vi "r3_Pick&Place_ladder_shih_v10_MPTv2.vi"() -> ()   [LabVIEW 2016]
uses:
  WTF is this.ctl
  Classes/Controllers/I-O/Copy of NI-DAQ Folder/NI-DAQ.lvclass
  D:/INTT/V1/Classes/Controllers/I-O/Copy of I-O Folder/I-O.lvclass
  Classes/Controllers/Dispenser/Copy of Ultimus V2 Folder/Ultimus V2.lvclass
  <vilib>/Analysis/coordinate.llb/2D Cartesian Coordinate Rotation (Scalar).vi
  <vilib>/Utility/file.llb/Read Delimited Spreadsheet (DBL).vi
  <vilib>/Utility/file.llb/Write Delimited Spreadsheet (DBL).vi
  Classes/Controllers/Motion/Copy of Motion Folder/Motion.lvclass
  Classes/Controllers/Camera/Copy of Controller Folder/Controller.lvclass
  <vilib>/Analysis/NI_AALPro.lvlib
  Classes/Controllers/I-O/Copy of I-O Folder/I-O.lvclass
panel:
  out "file indicator":dbl[][](array[numeric])
  out "?":dbl[](array[numeric]) format="%#_8g"
  in  "offset":dbl[](array[numeric])=[0.0, 0.0, 0.0, 0.0] format="%#_8g"
  out "HDI center positions":dbl[][](array[numeric]) format="%#_8g"
  out "HDI center positions":dbl[][](array[numeric])=[[459.92445114002015, 980.2358762511564, 78.77350133595746, 0.0015214873297426886]] format="%#_8g"
  out "CT sum up":dbl[](array[numeric])
  in  "txt switch":bool
  in  "MPT offset":dbl[][](array[numeric])=[[0.0, 0.0, 0.0, 0.0], [0.0, 0.0, 0.0, 0.0]] format="%#_8g"
  out "CT HPoS":dbl[][](array[numeric]) format="%#_8g"
  out "chip distance by OGP":dbl format="%#_8g"
  out "displacement":dbl[](array[numeric])
  out "gantry position test":dbl[](array[numeric])
  out "gantry target position":dbl[](array[numeric])
  out "chip distance by gantry":dbl format="%#_8g"
  out "after SL":dbl[](array[numeric]) format="%#_8g"
  out "after SR":dbl[](array[numeric]) format="%#_8g"
  out "after NL":dbl[](array[numeric]) format="%#_8g"
  out "S chip":dbl[](array[numeric]) format="%#_8g"
  out "N chip":dbl[](array[numeric]) format="%#_8g"
  in  "?":path=path "C:/Users/PAGANIS/Desktop/shih cheng wei/OGP/test1-2.txt"
  out "bless from OGP !!! Center of  stave":dbl[](array[numeric])
  out "bless from OGP !! measured stave size":dbl[](array[numeric])
  in  "Bless from OGP":bool
  out "FROM Detail !!! Center of module on stave":dbl[](array[numeric])
  out "FROM Detail !! measured stave size":dbl[](array[numeric])
  in  "Align Stave in detail":bool
  in  "check height?":bool=TRUE
  in  "Uttimus presssure":i64=10
  out "Status":bool
  out "measured HDI top-left position":dbl[][](array[numeric])
  in  "HDI vacuum channel":i32=18
  in  "vacuum":bool=TRUE
  in  "HDI vacuum":bool
  out "measured stave size":dbl[](array[numeric])
  out "Stave mark":dbl[][](array[numeric])
  out "Center of module on stave":dbl[](array[numeric])
  out "Measured HDI size":dbl[][](array[numeric])
  out "MPT positions on stave":T1[][](array[typedef]) format="%#_8g"
  in  "Default Stave dimension":dbl[](array[numeric])=[34.0, 472.0, -0.335295, -0.000320234]
  in  "Default Stave upper left mark":dbl[](array[numeric])=[584.376, 675.576, 70.9882, 0.000840064]
  out "Needle parking position":dbl[](array[numeric])
  in  "Uppler / Lower Stave":bool=TRUE
  out "Gantry current position":dbl[](array[numeric])
  in  "READ Position":bool
  in  "Needle Height Compenstation\n(glue gap)":dbl=0.33
  in  "Needle Alignment":bool
  in  "Parking position":dbl[](array[numeric])=[625.0, 625.0, 0.0, 0.01]
  in  "GOTO":bool
  in  "Default Pickup Tool Position":dbl[][](array[numeric])=[[166.21919, 608.63665, 49.475503, -0.0151898], [700.0, 800.0, 20.0, 0.01]]
  in  "deposit glue module":i32=1
  in  "Default HDI alignment \nmark position":dbl[](array[numeric])=[139.81, 893.561, 78.9867, 0.000191129]
  in  "Default HDI size":dbl[](array[numeric])=[24.2437, 231.446, -0.099339, 0.000191129]
  out "# of tasks excuted":i32
  out "PickupTool \nCenterPosition":dbl[](array[numeric]) format="%#_8g"
  in  "Inititalize":bool
  in  "Pick and place":bool
  in  "Deposit Glue":bool
  in  "Measure Pickup Tools":bool
  in  "Align Stave":bool
  out "default module position on stave":dbl[][](array[numeric])
  in  "Stop":bool
  in  "Measure HDI":bool
  # "Ladder Assembly"
  # "To switch the north/south\ntxt file \nswitch \noffset\nmodule pick up tool\nmodule direction"
  # "upper : north \nlower : south"
  # "Upper\nmodule"
  # "Lower\nmodule"
  # "Sensor 0.32 -> 200 micron glue thickness\nChips 0.37-> 140 micron glue thickness"
  # "ACTIONS"
  # "theta had *-1"
  # "Pick up tool and needle"
  # "Module infomation"
  # "Pick and Place"
  # "after assembly"
  # "CT"
  # "+"
  # "+"
  # "="
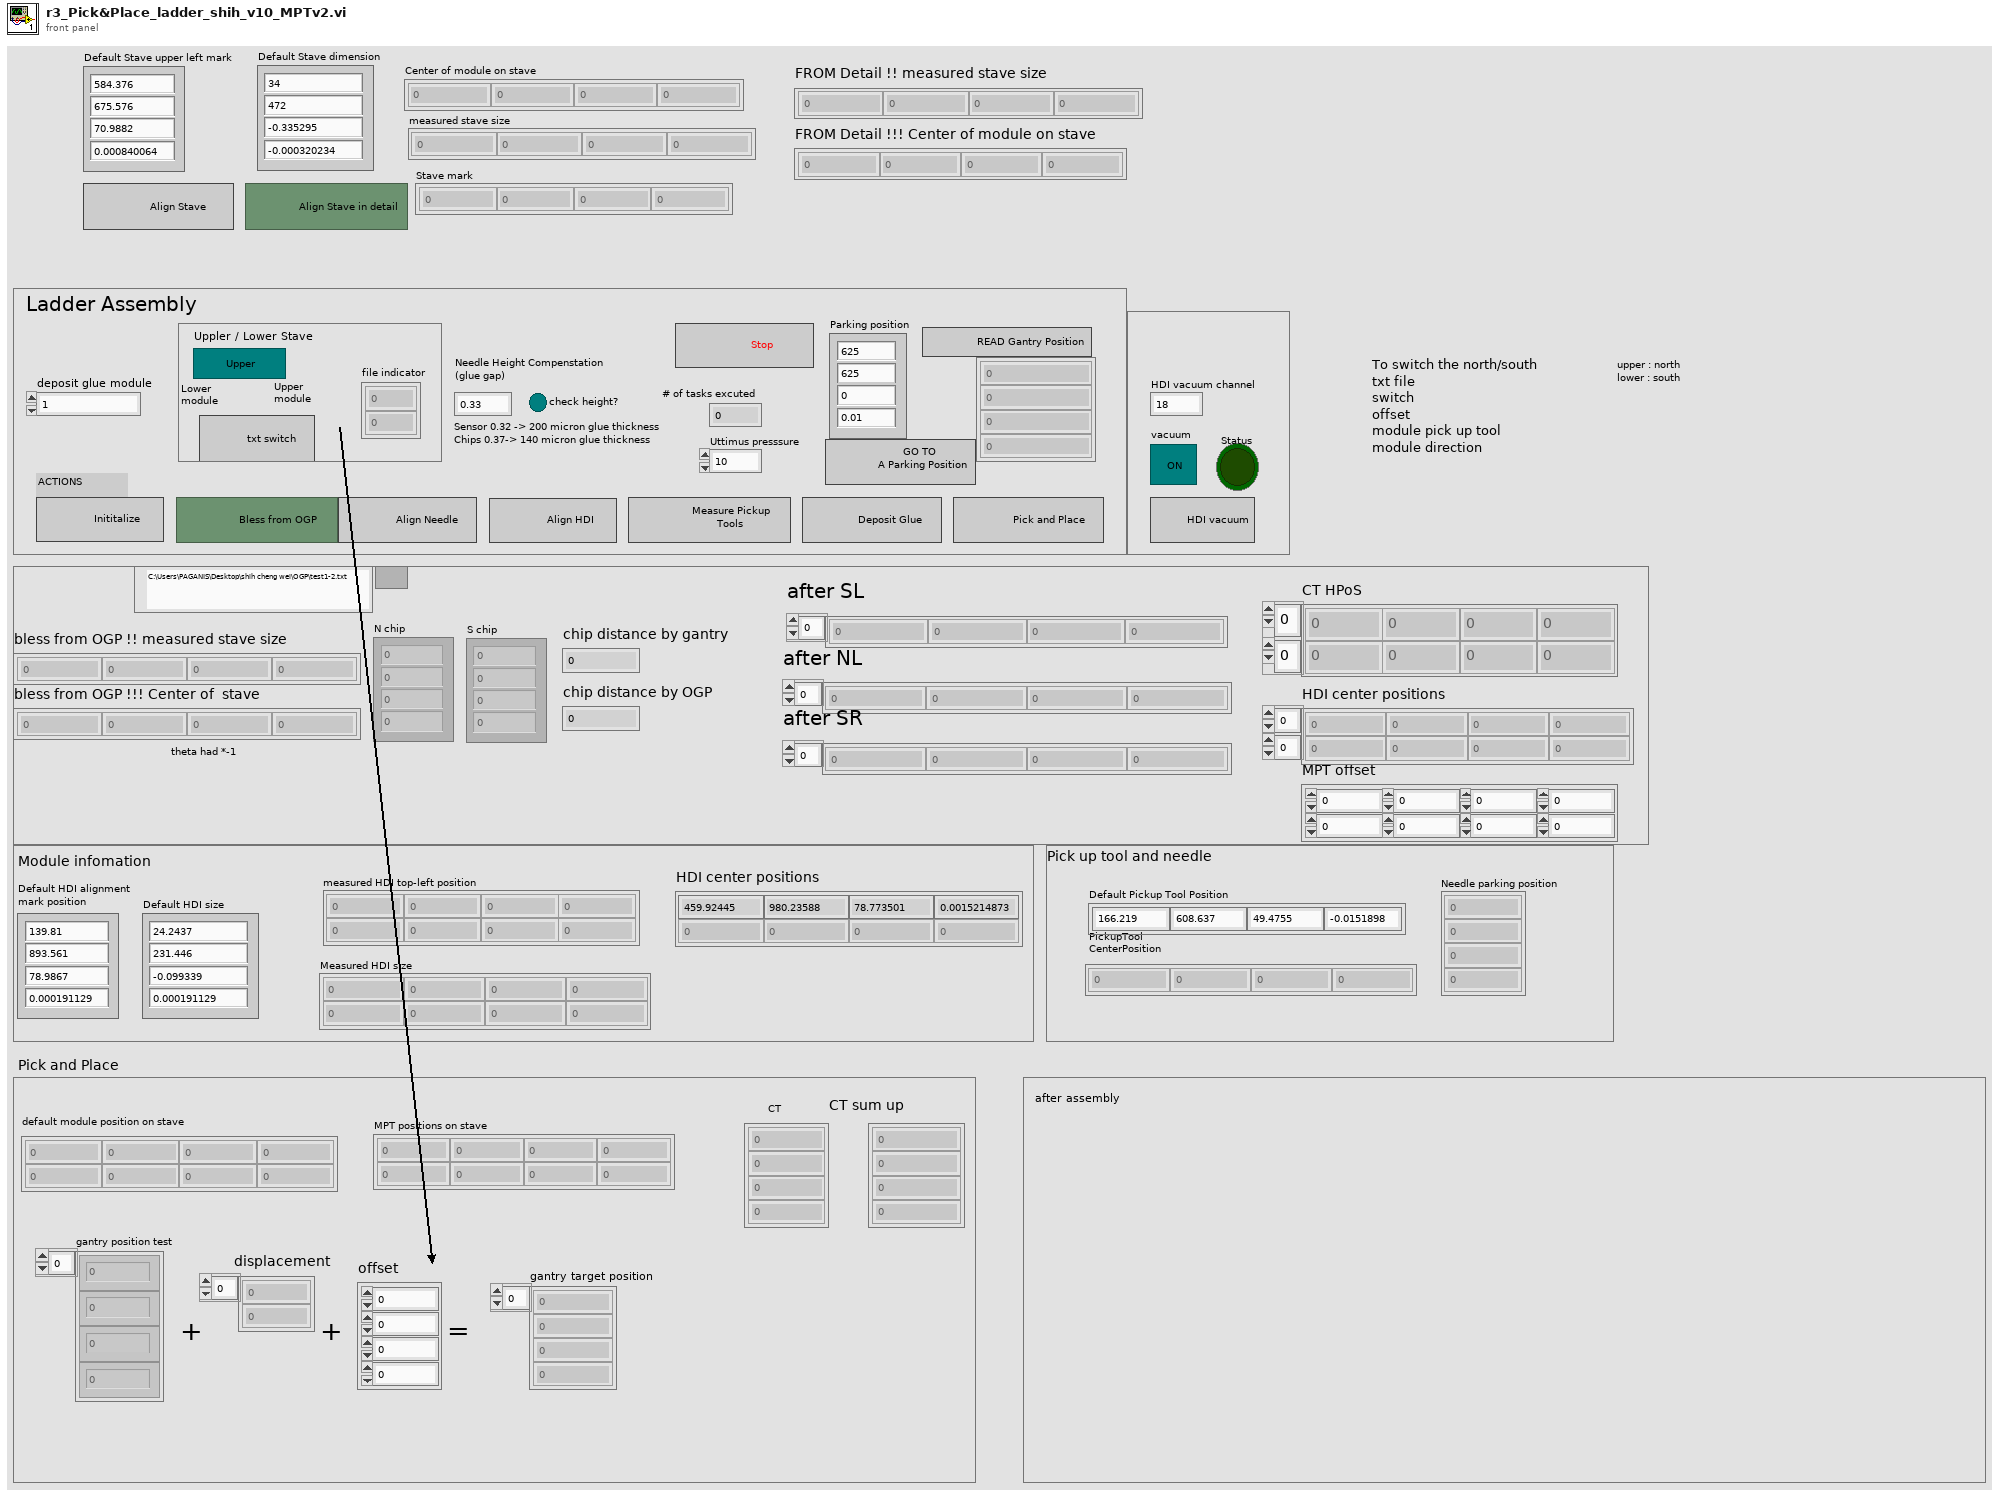
[diagram p1: front panel]
types:
  T1 = typedef "WTF is this.ctl" = dbl
  T2 = typedef "Controller.lvclass/Controllers.ctl" = cluster{"Copy of Motion.lvclass":refnum<class "Motion.lvclass">, "Copy of I-O.lvclass":refnum<class "I-O.lvclass">, "Copy of Dispenser.lvclass":refnum<class "Dispenser.lvclass">}
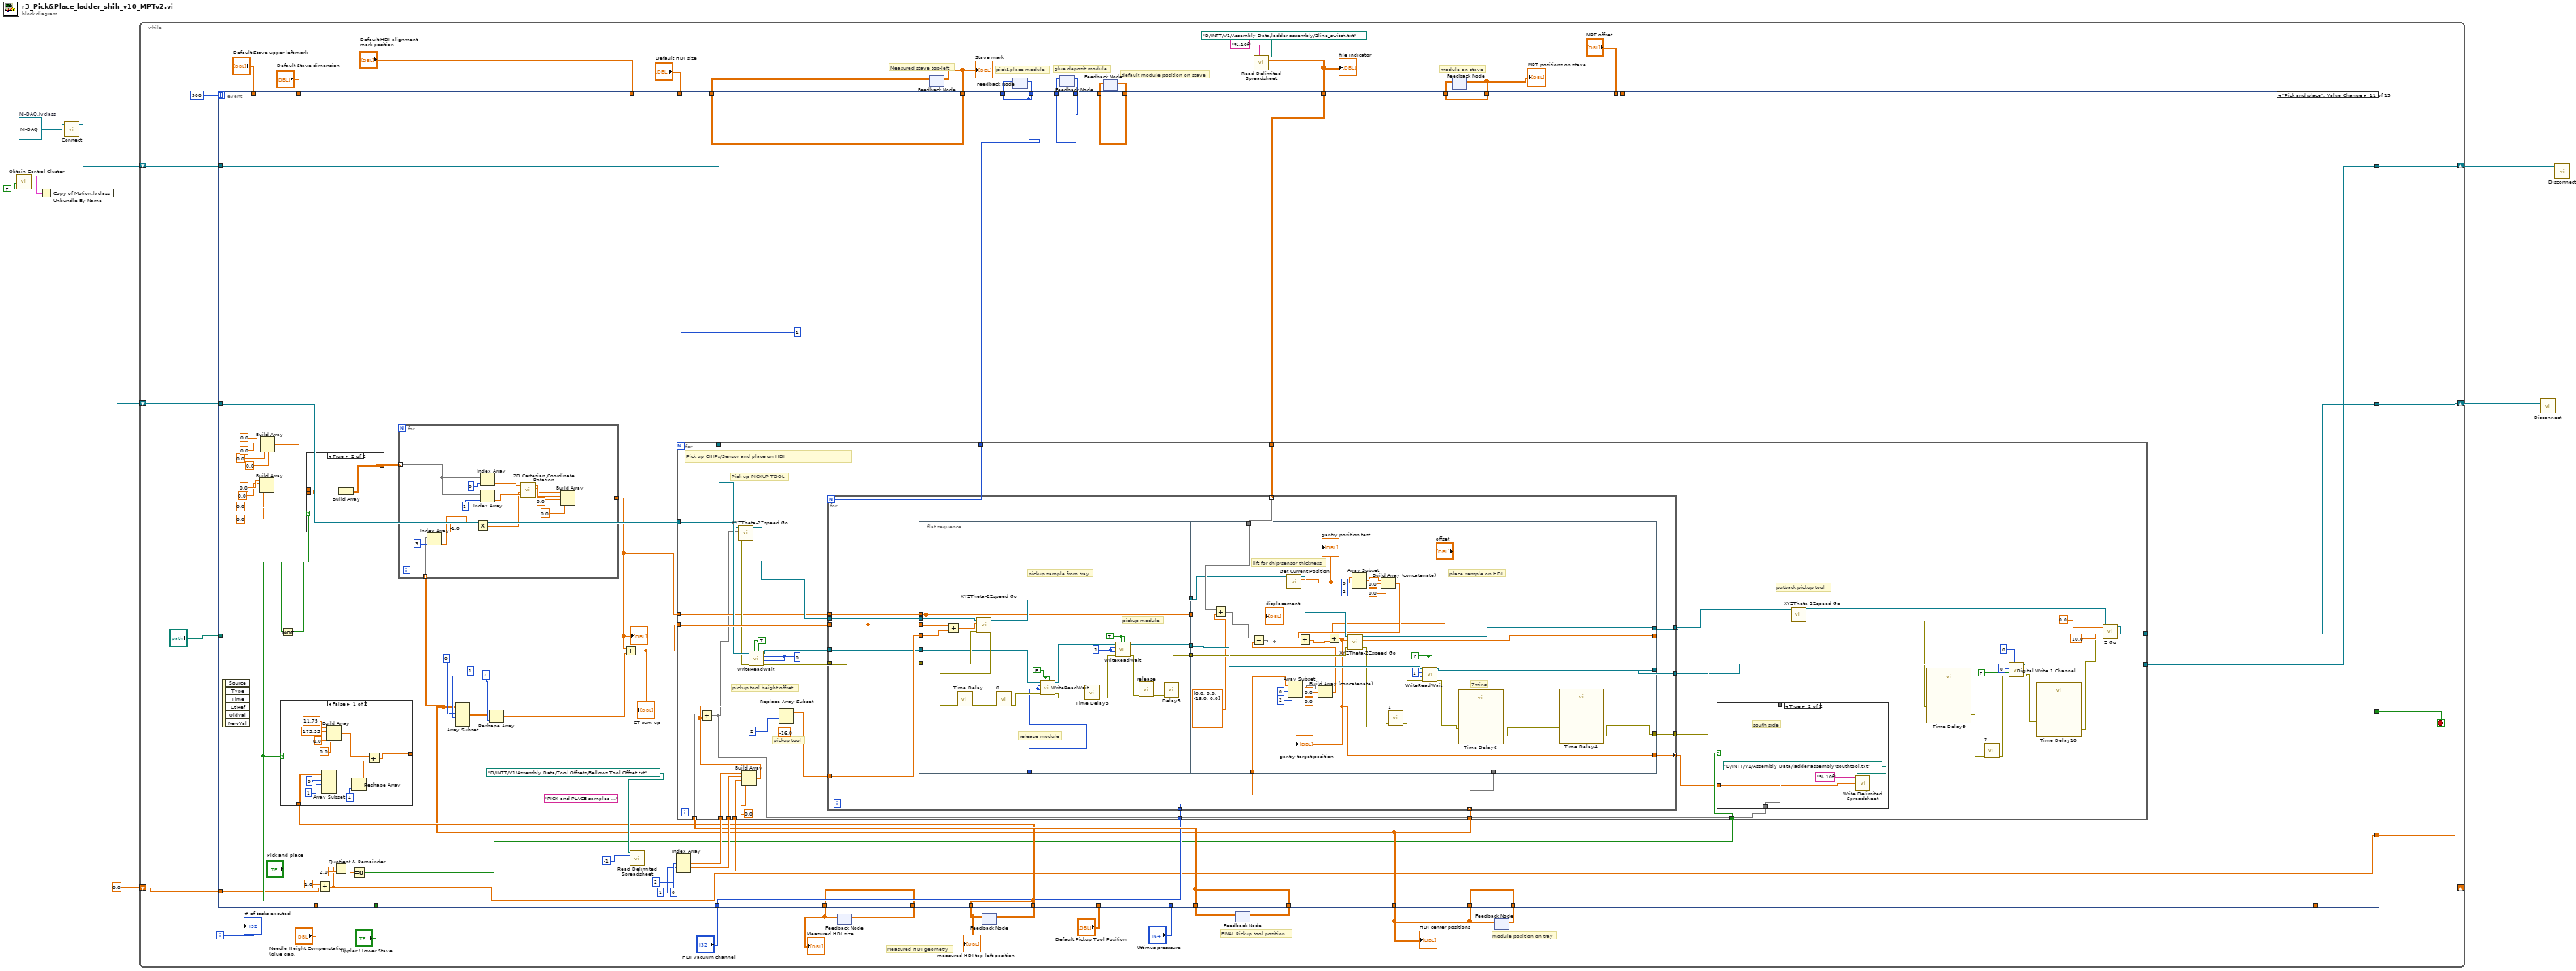
[diagram p0: block diagram]
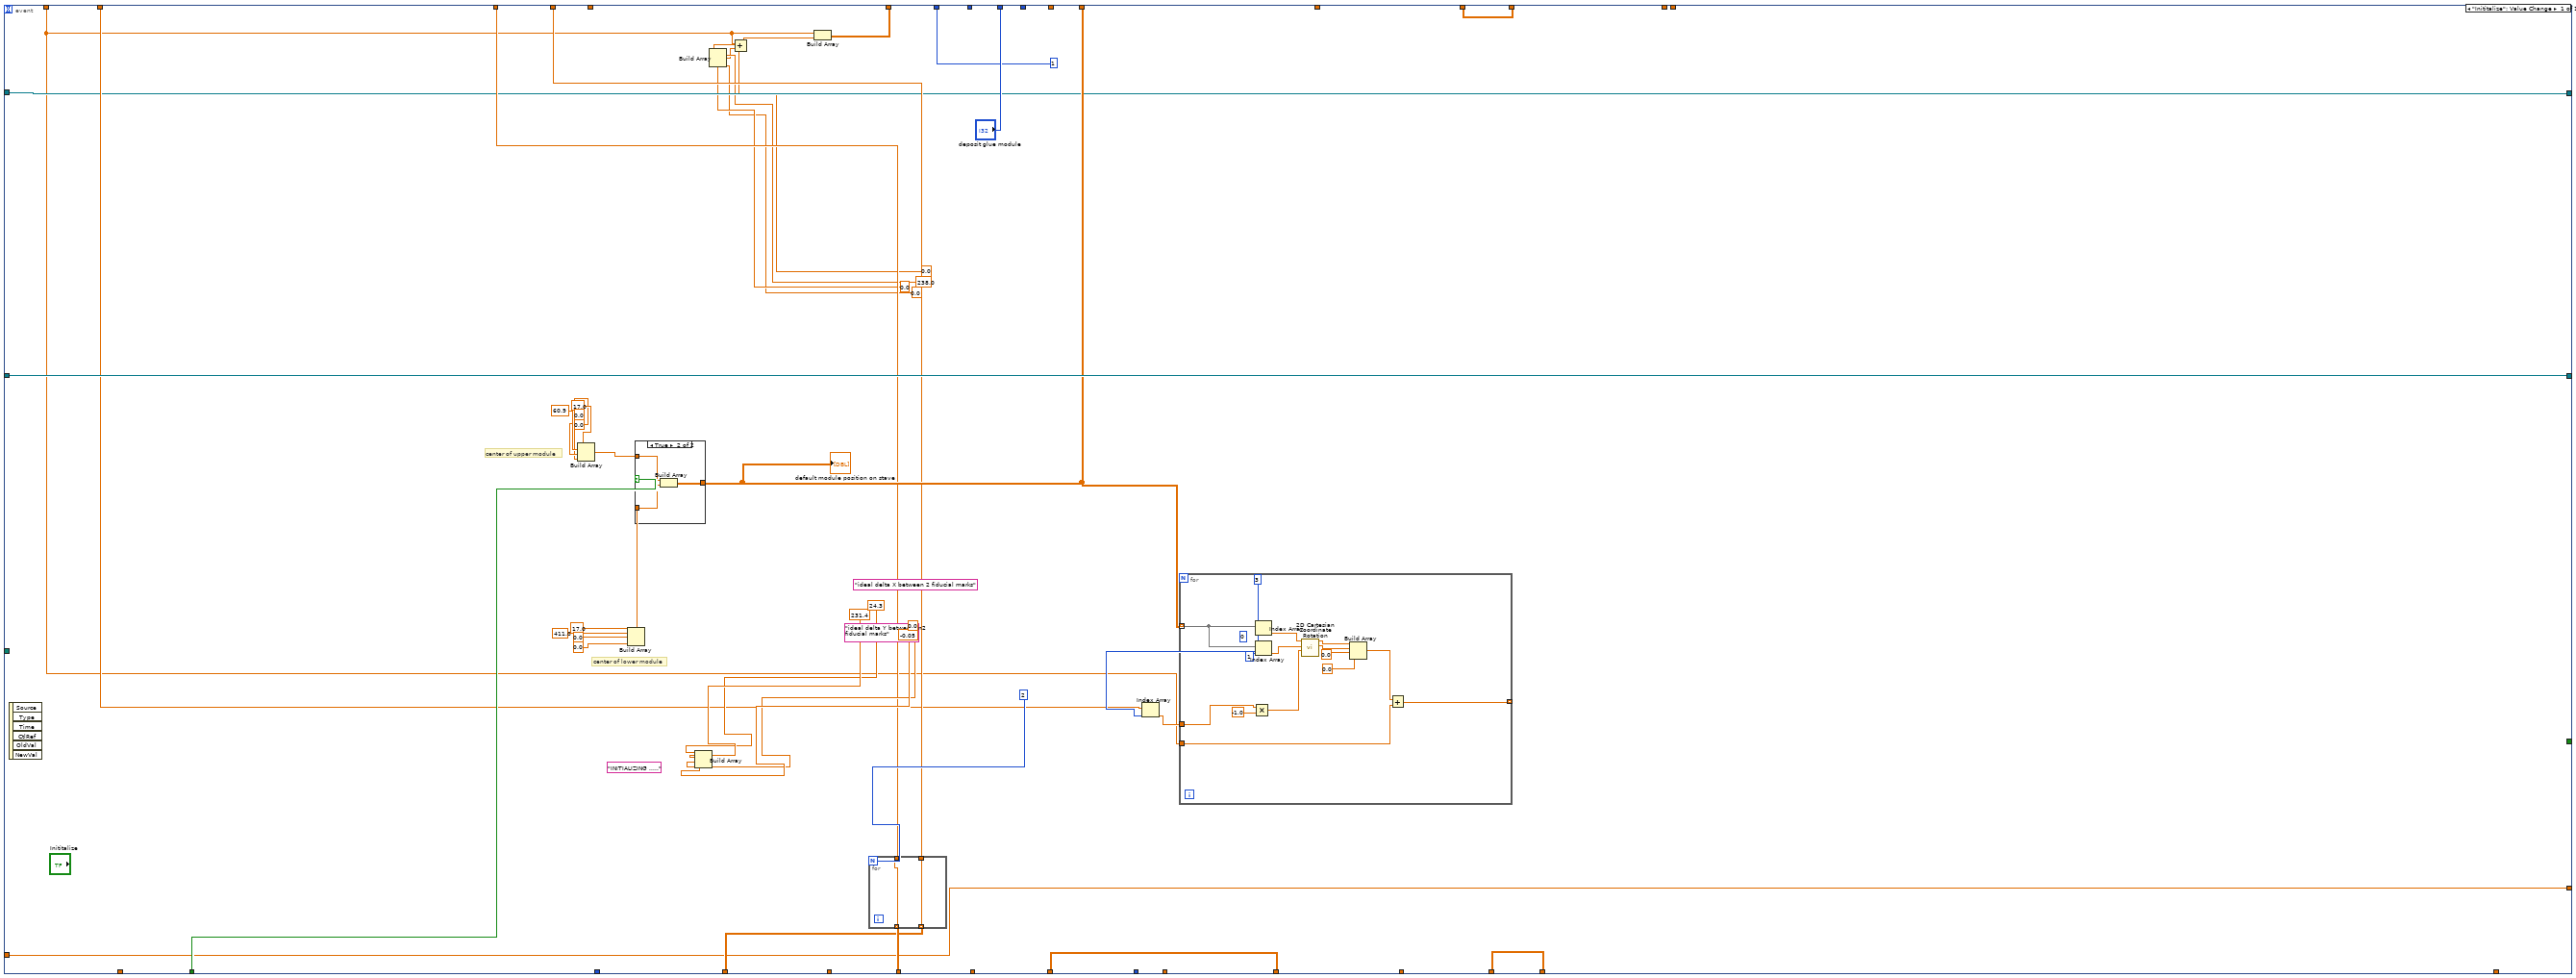
[diagram p2: hidden frame]
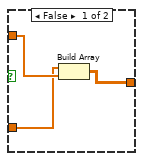
[diagram p3: hidden frame]
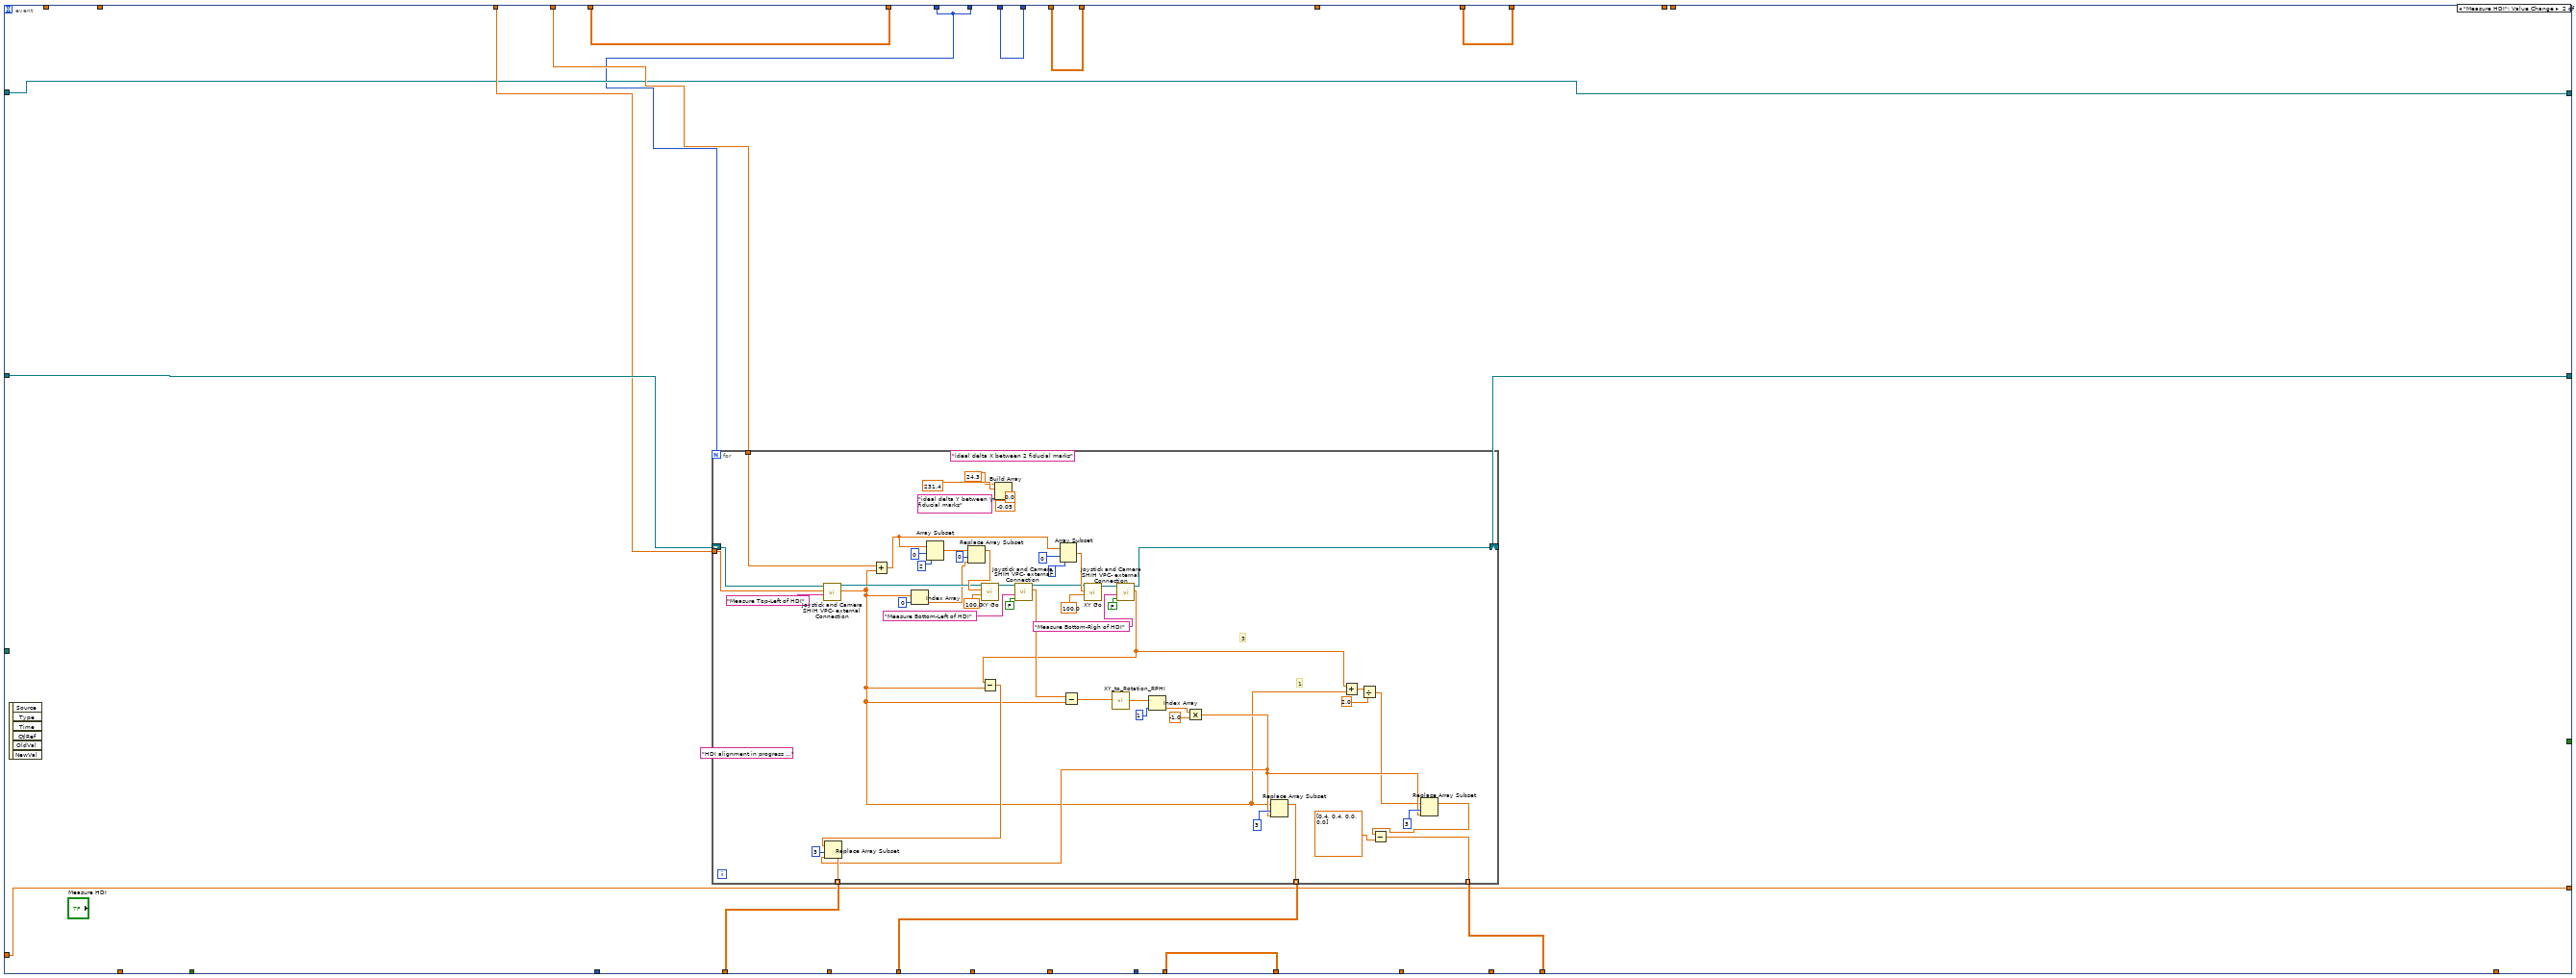
[diagram p4: hidden frame]
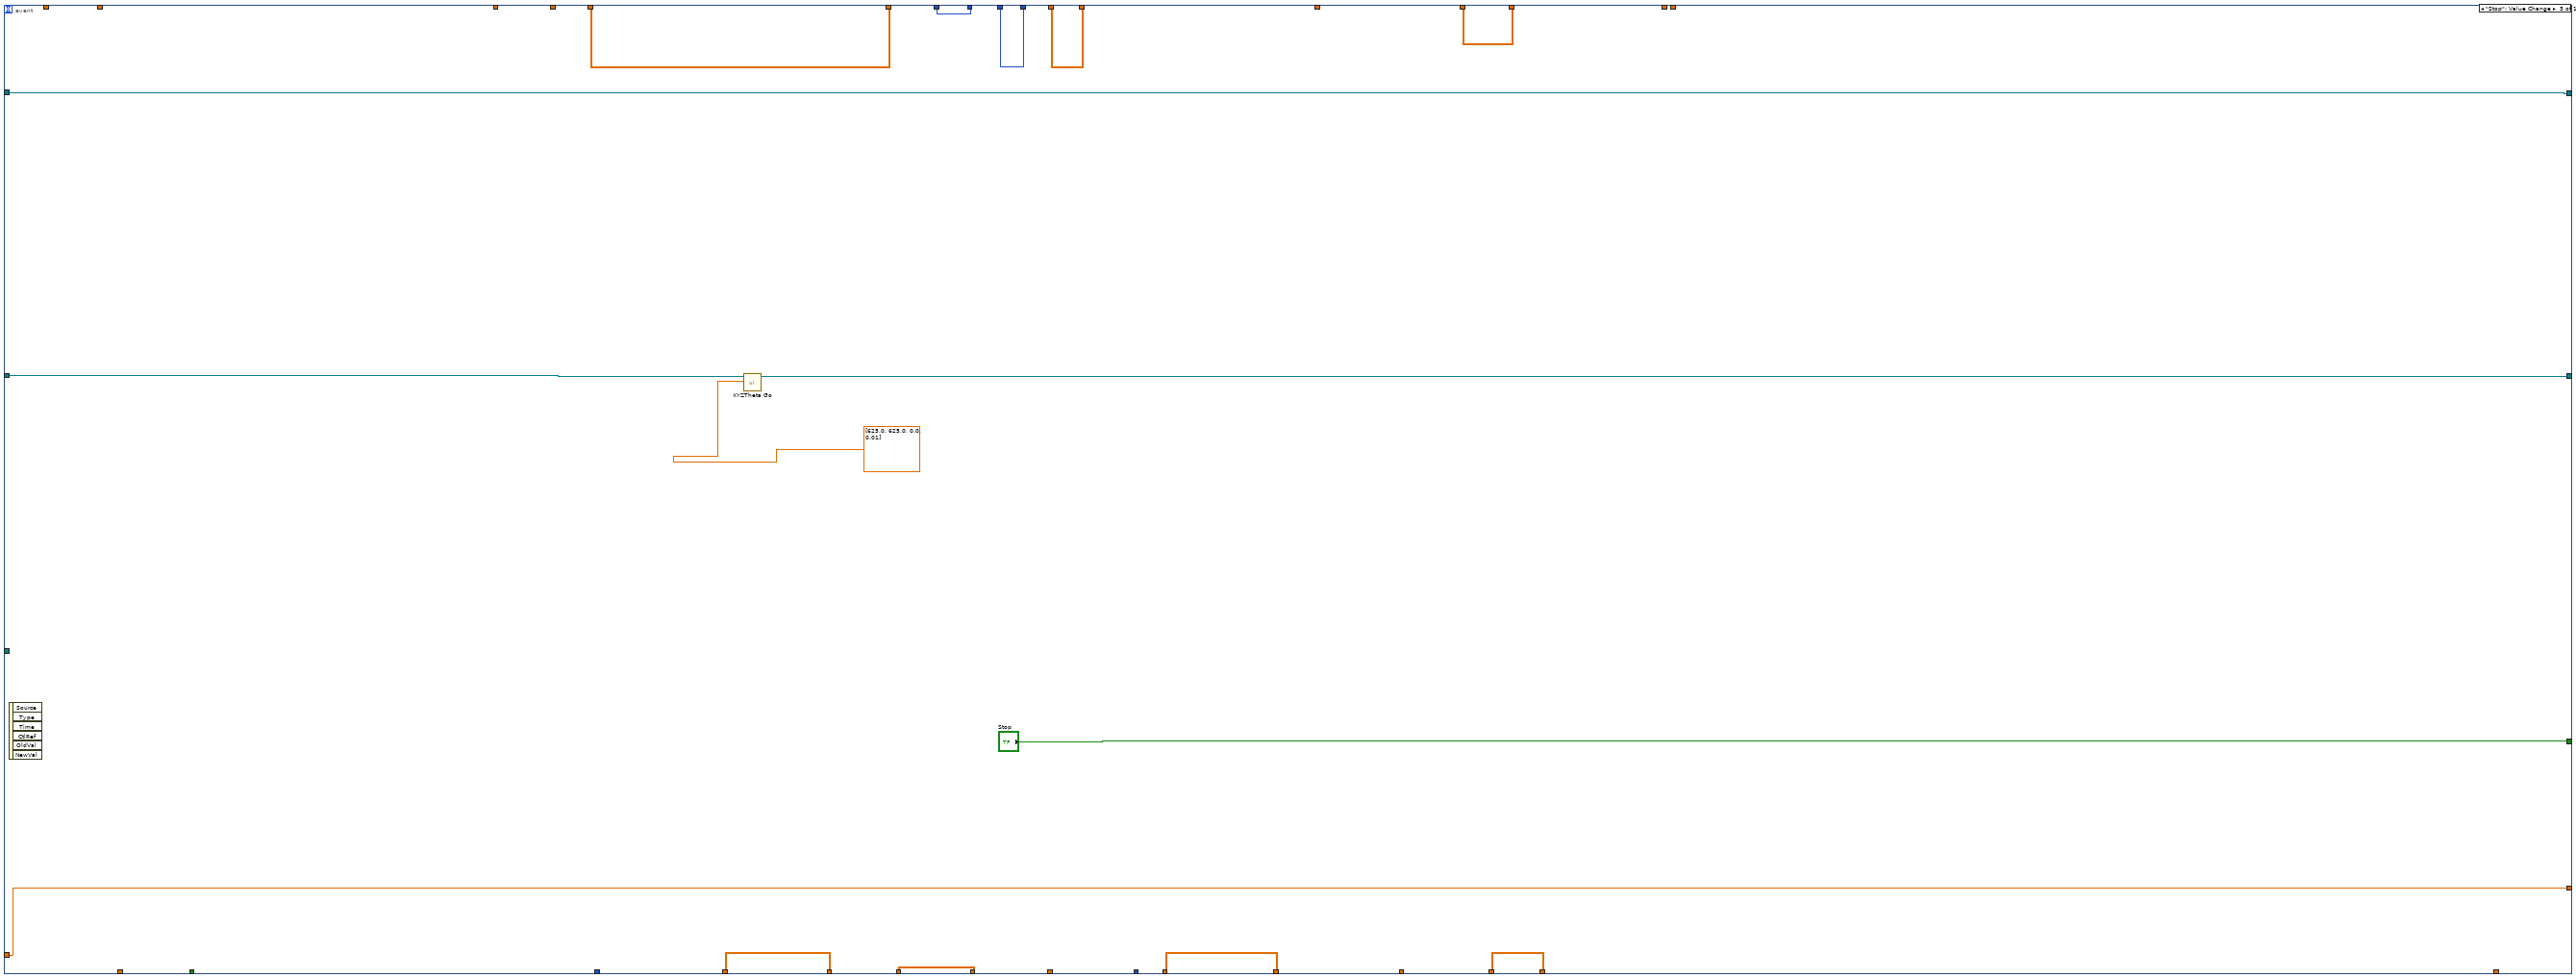
[diagram p5: hidden frame]
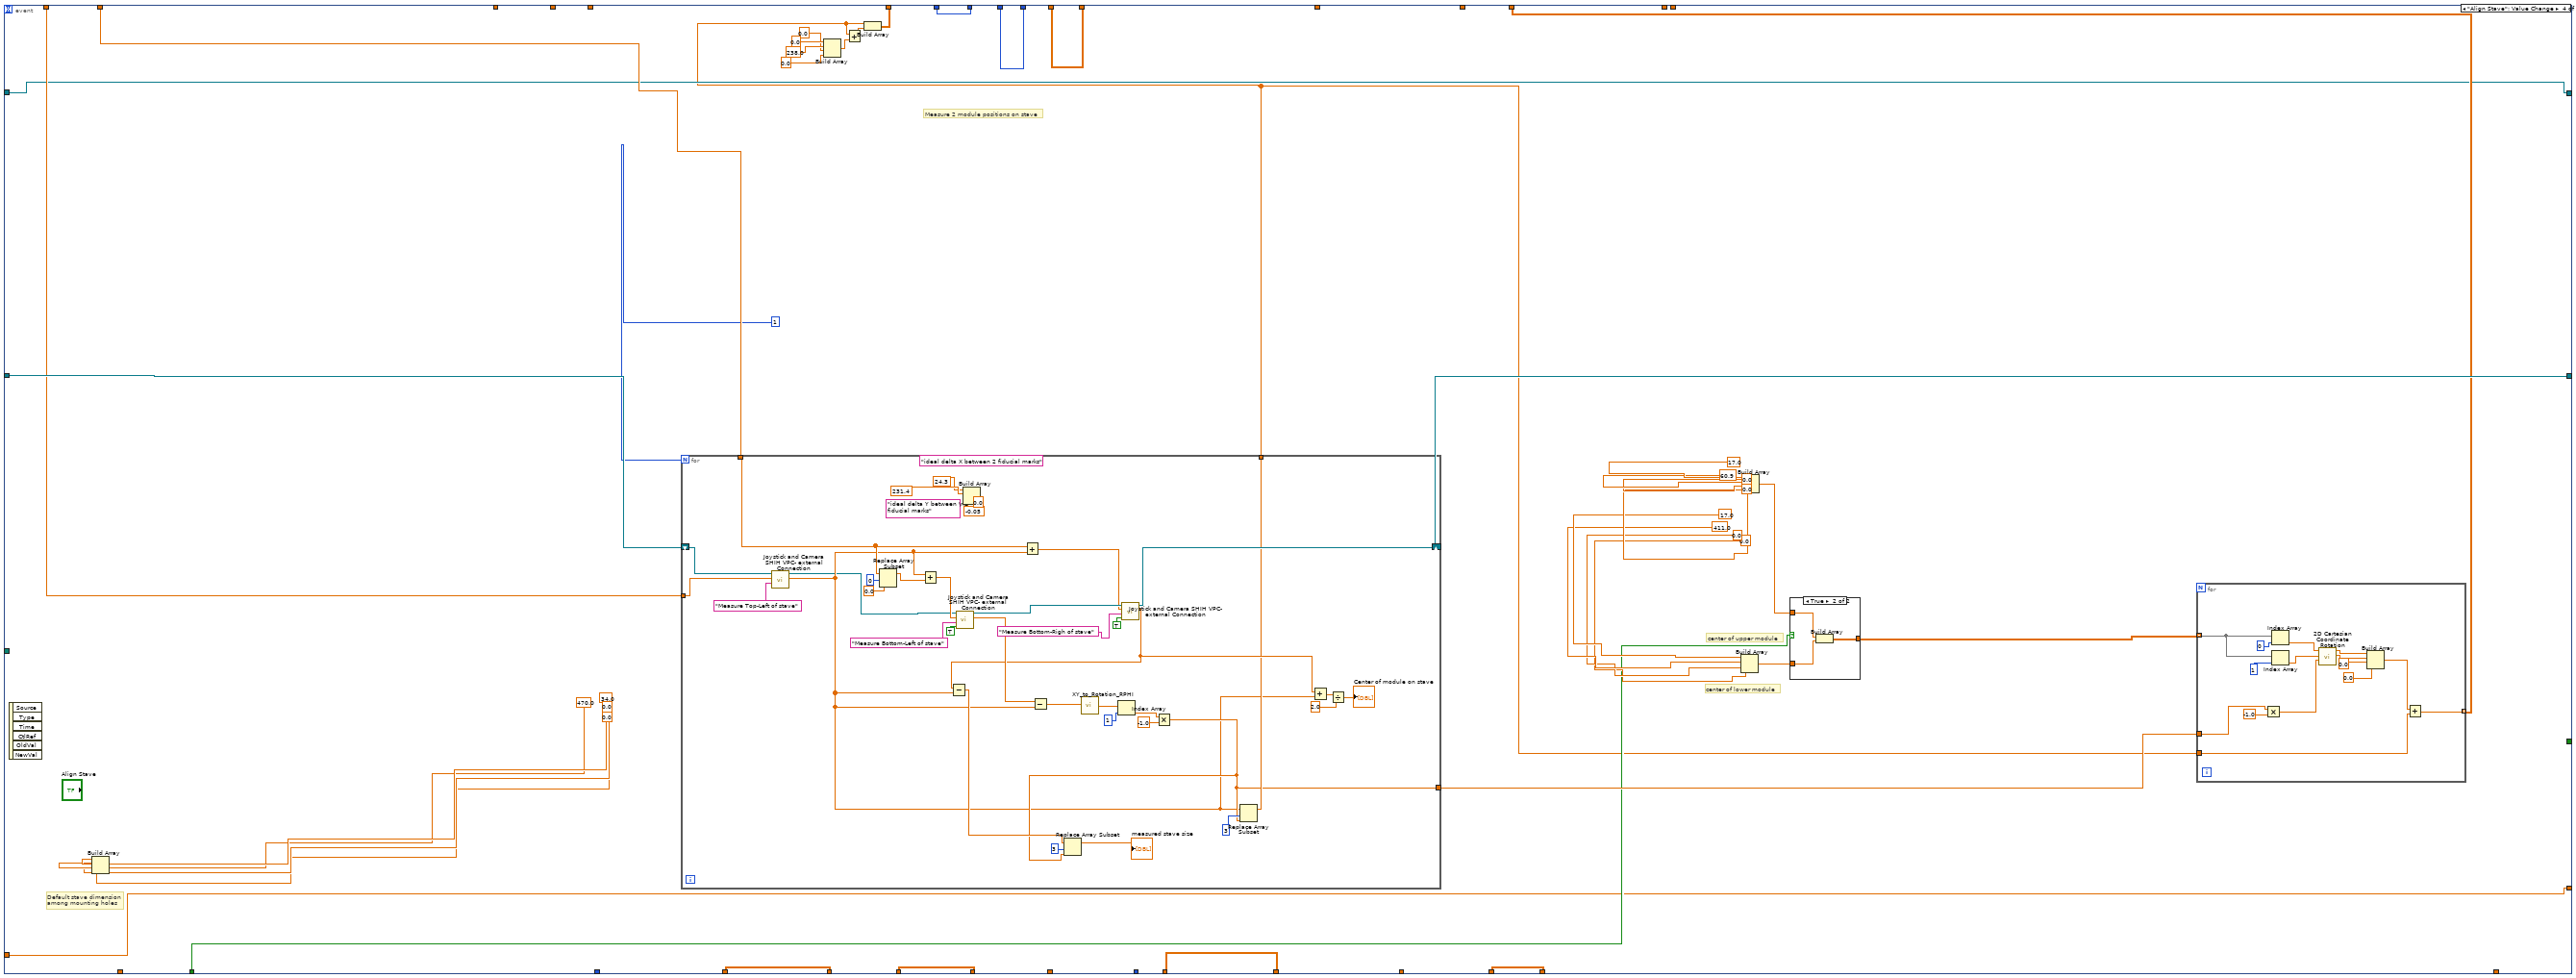
[diagram p6: hidden frame]
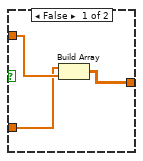
[diagram p7: hidden frame]
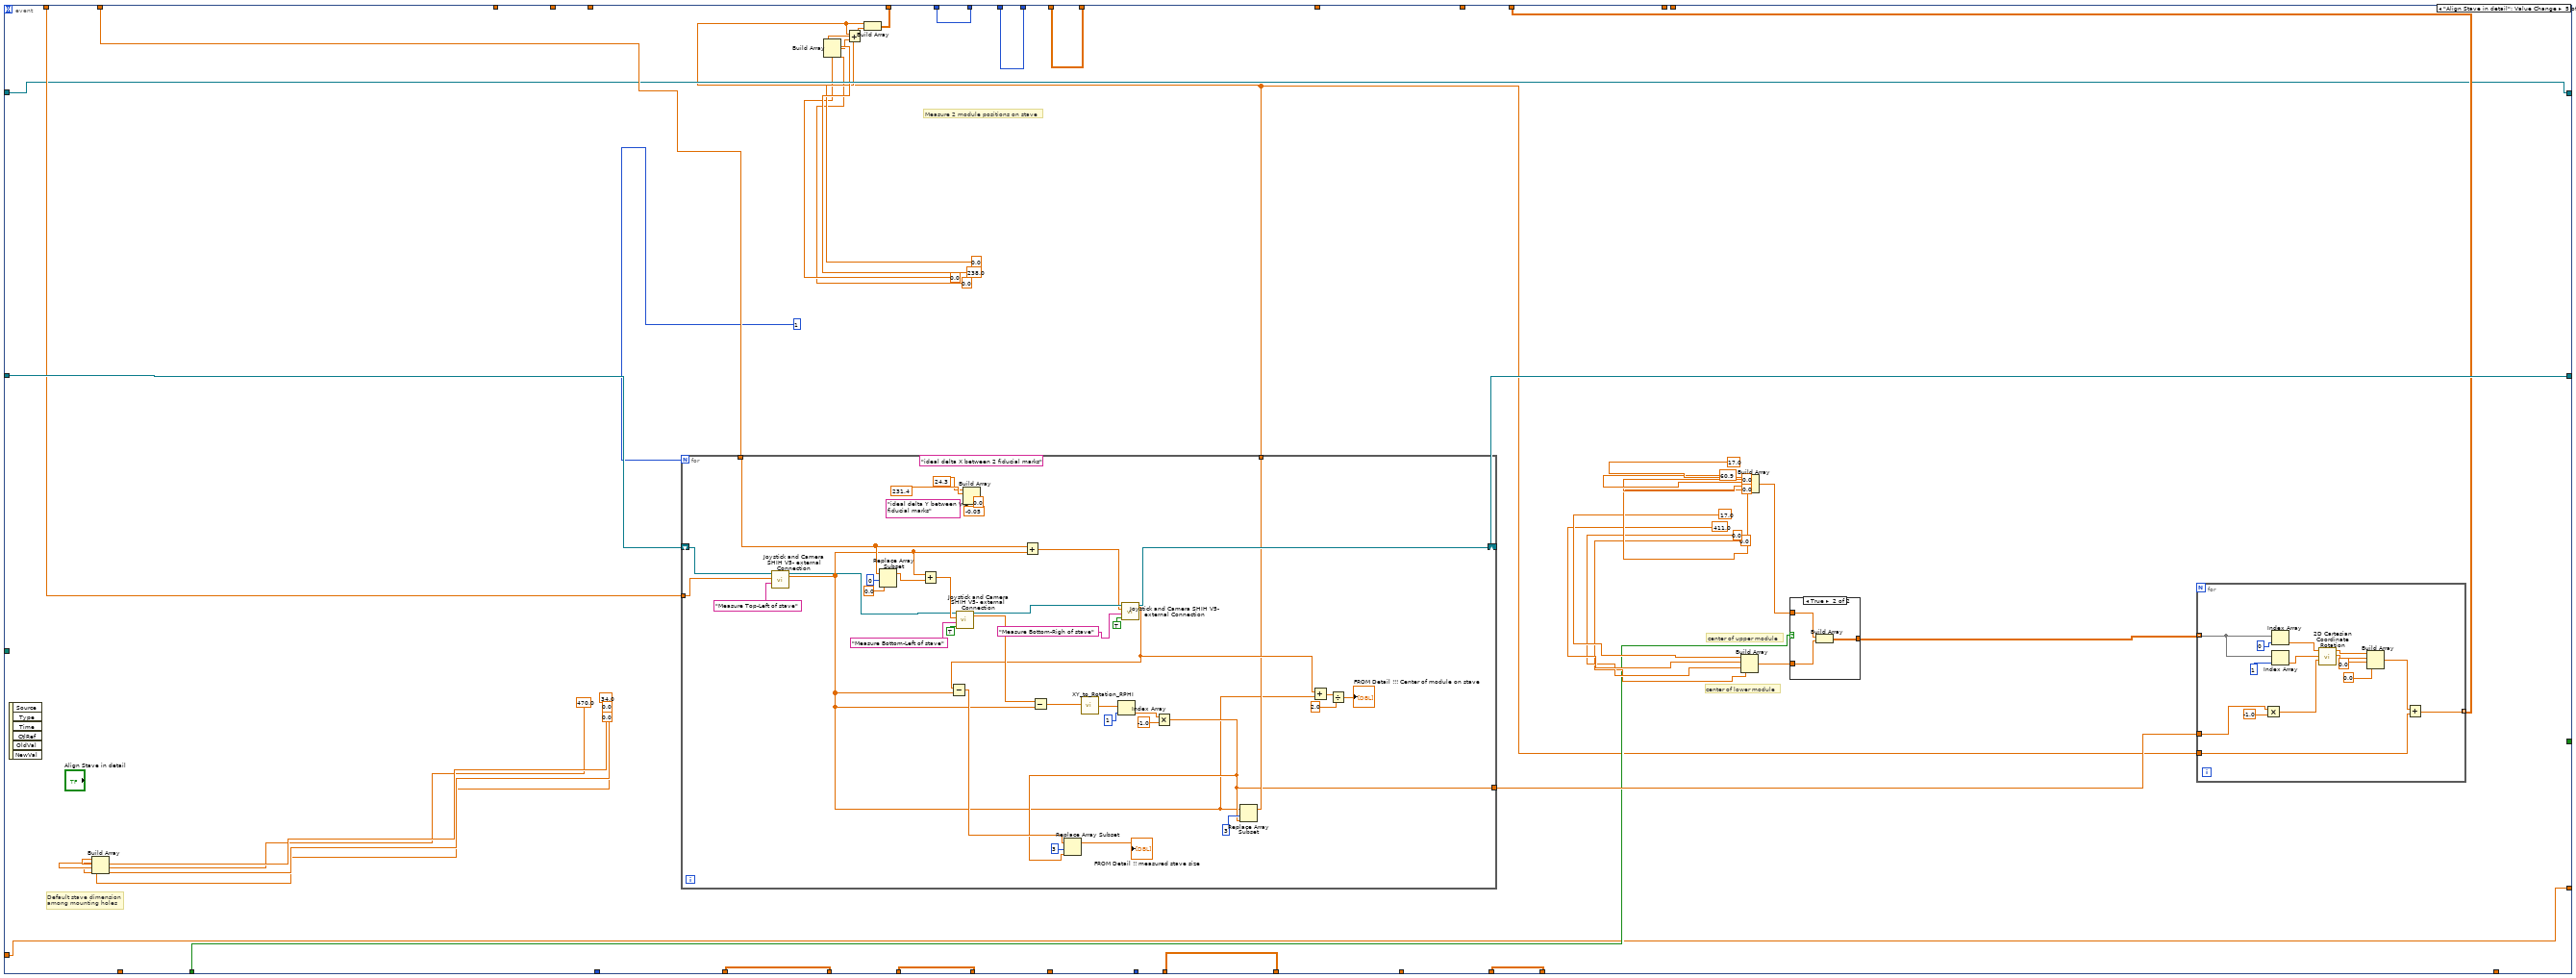
[diagram p8: hidden frame]
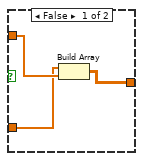
[diagram p9: hidden frame]
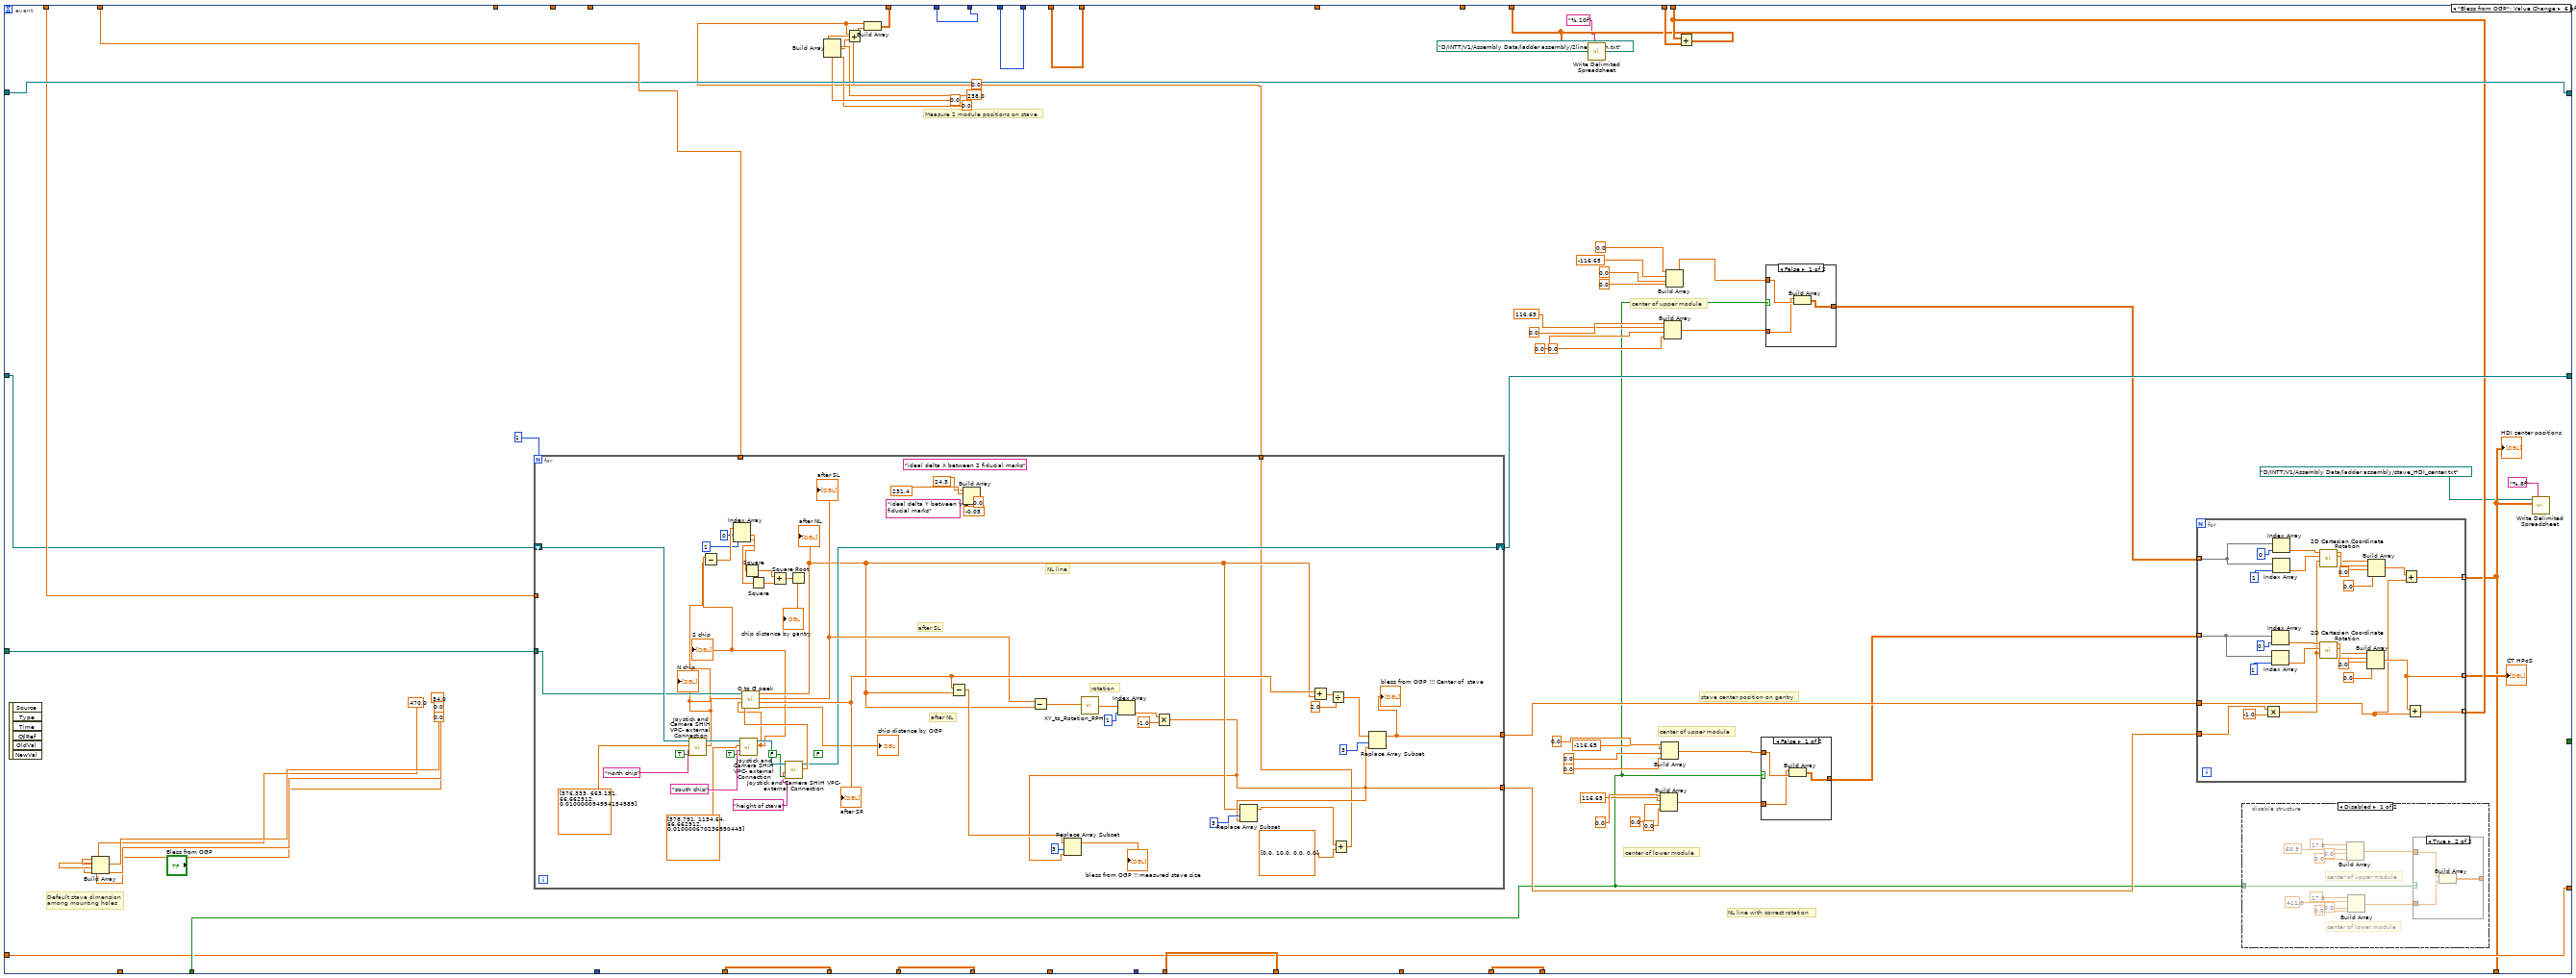
[diagram p10: hidden frame]
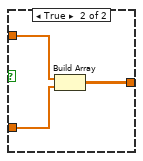
[diagram p11: hidden frame]
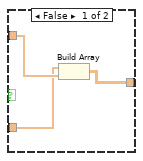
[diagram p12: hidden frame]
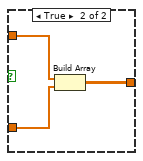
[diagram p14: hidden frame]
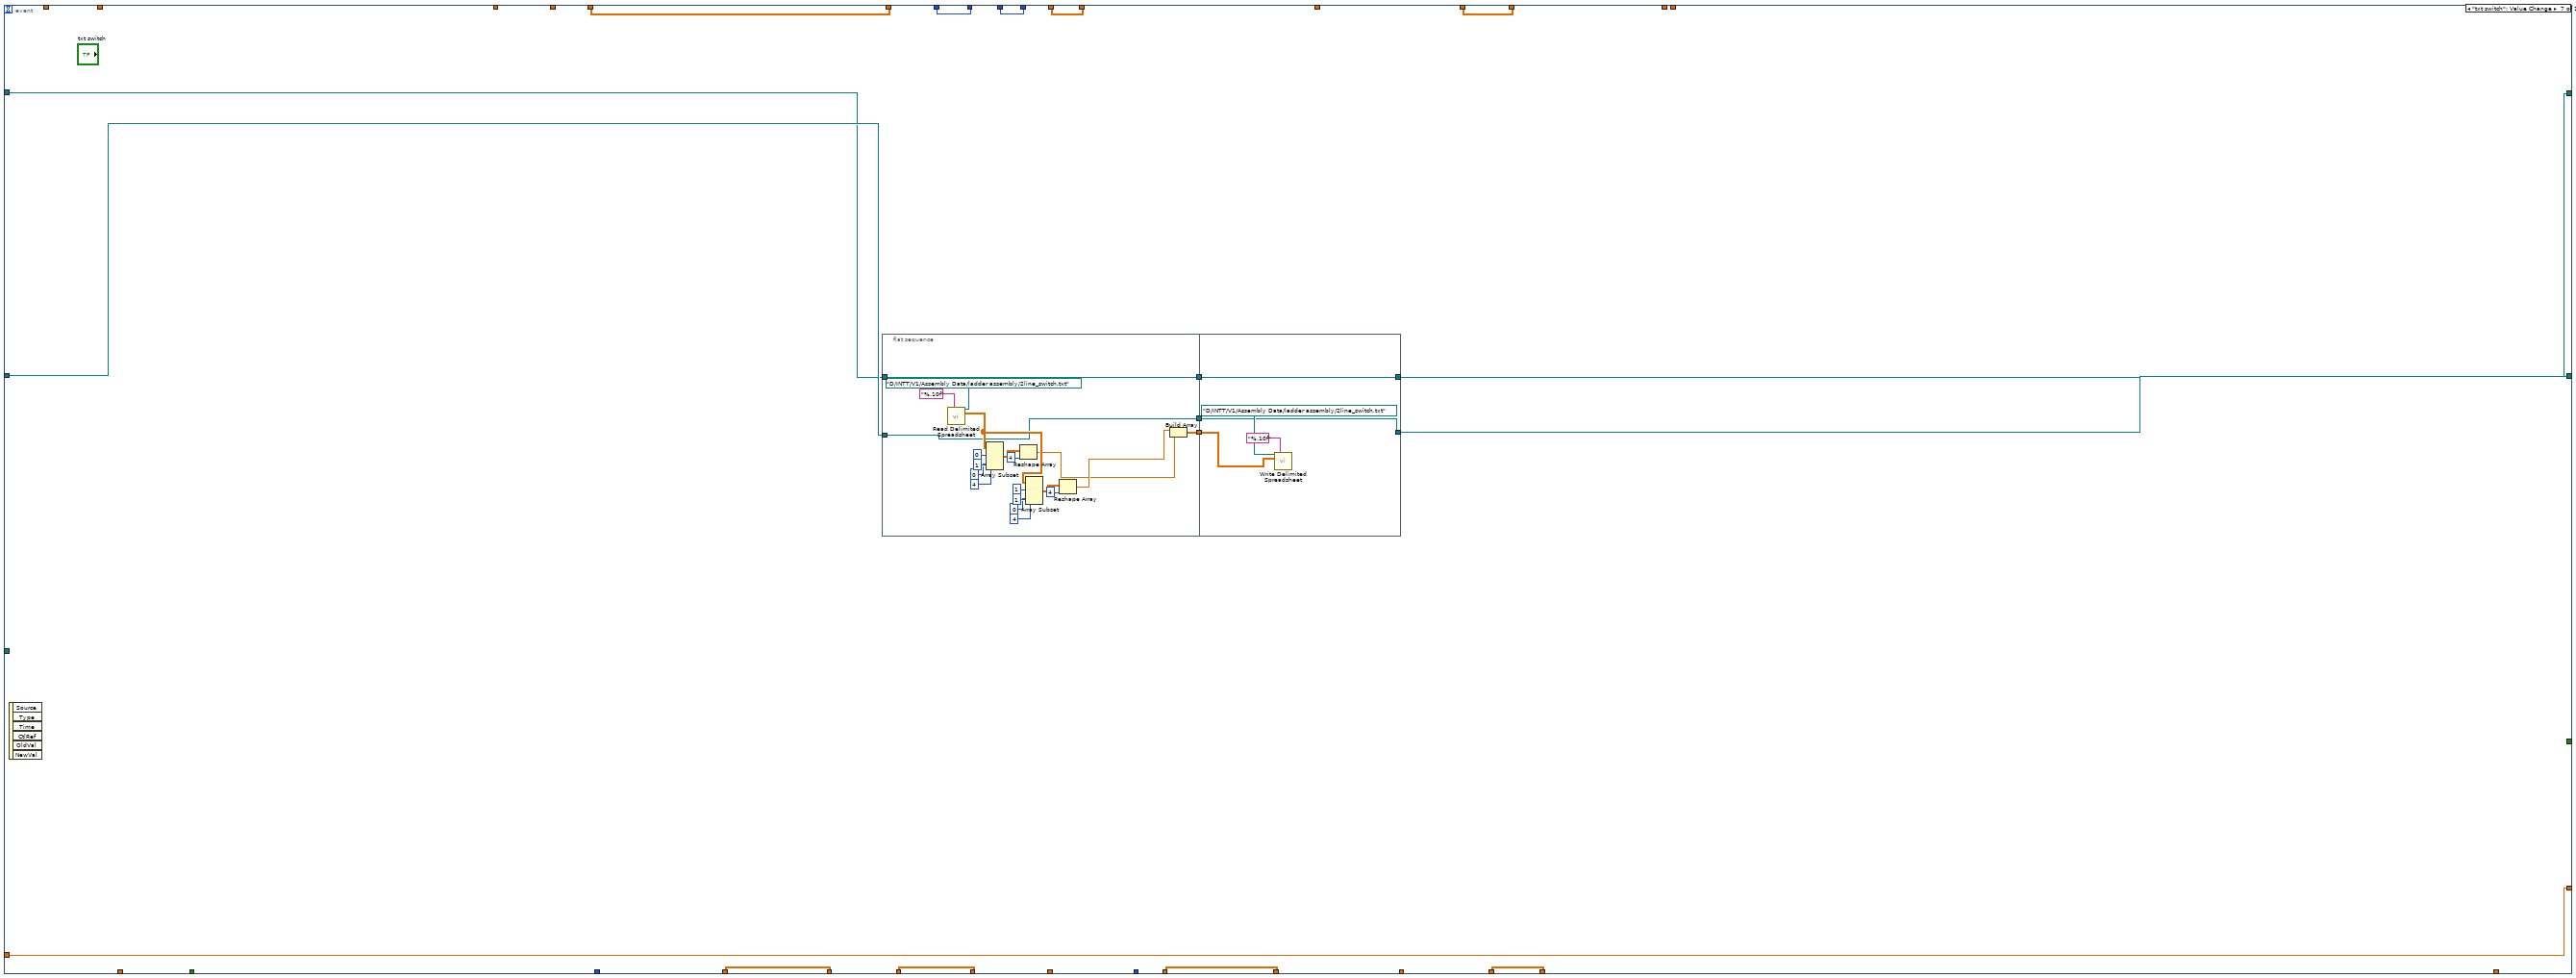
[diagram p15: hidden frame]
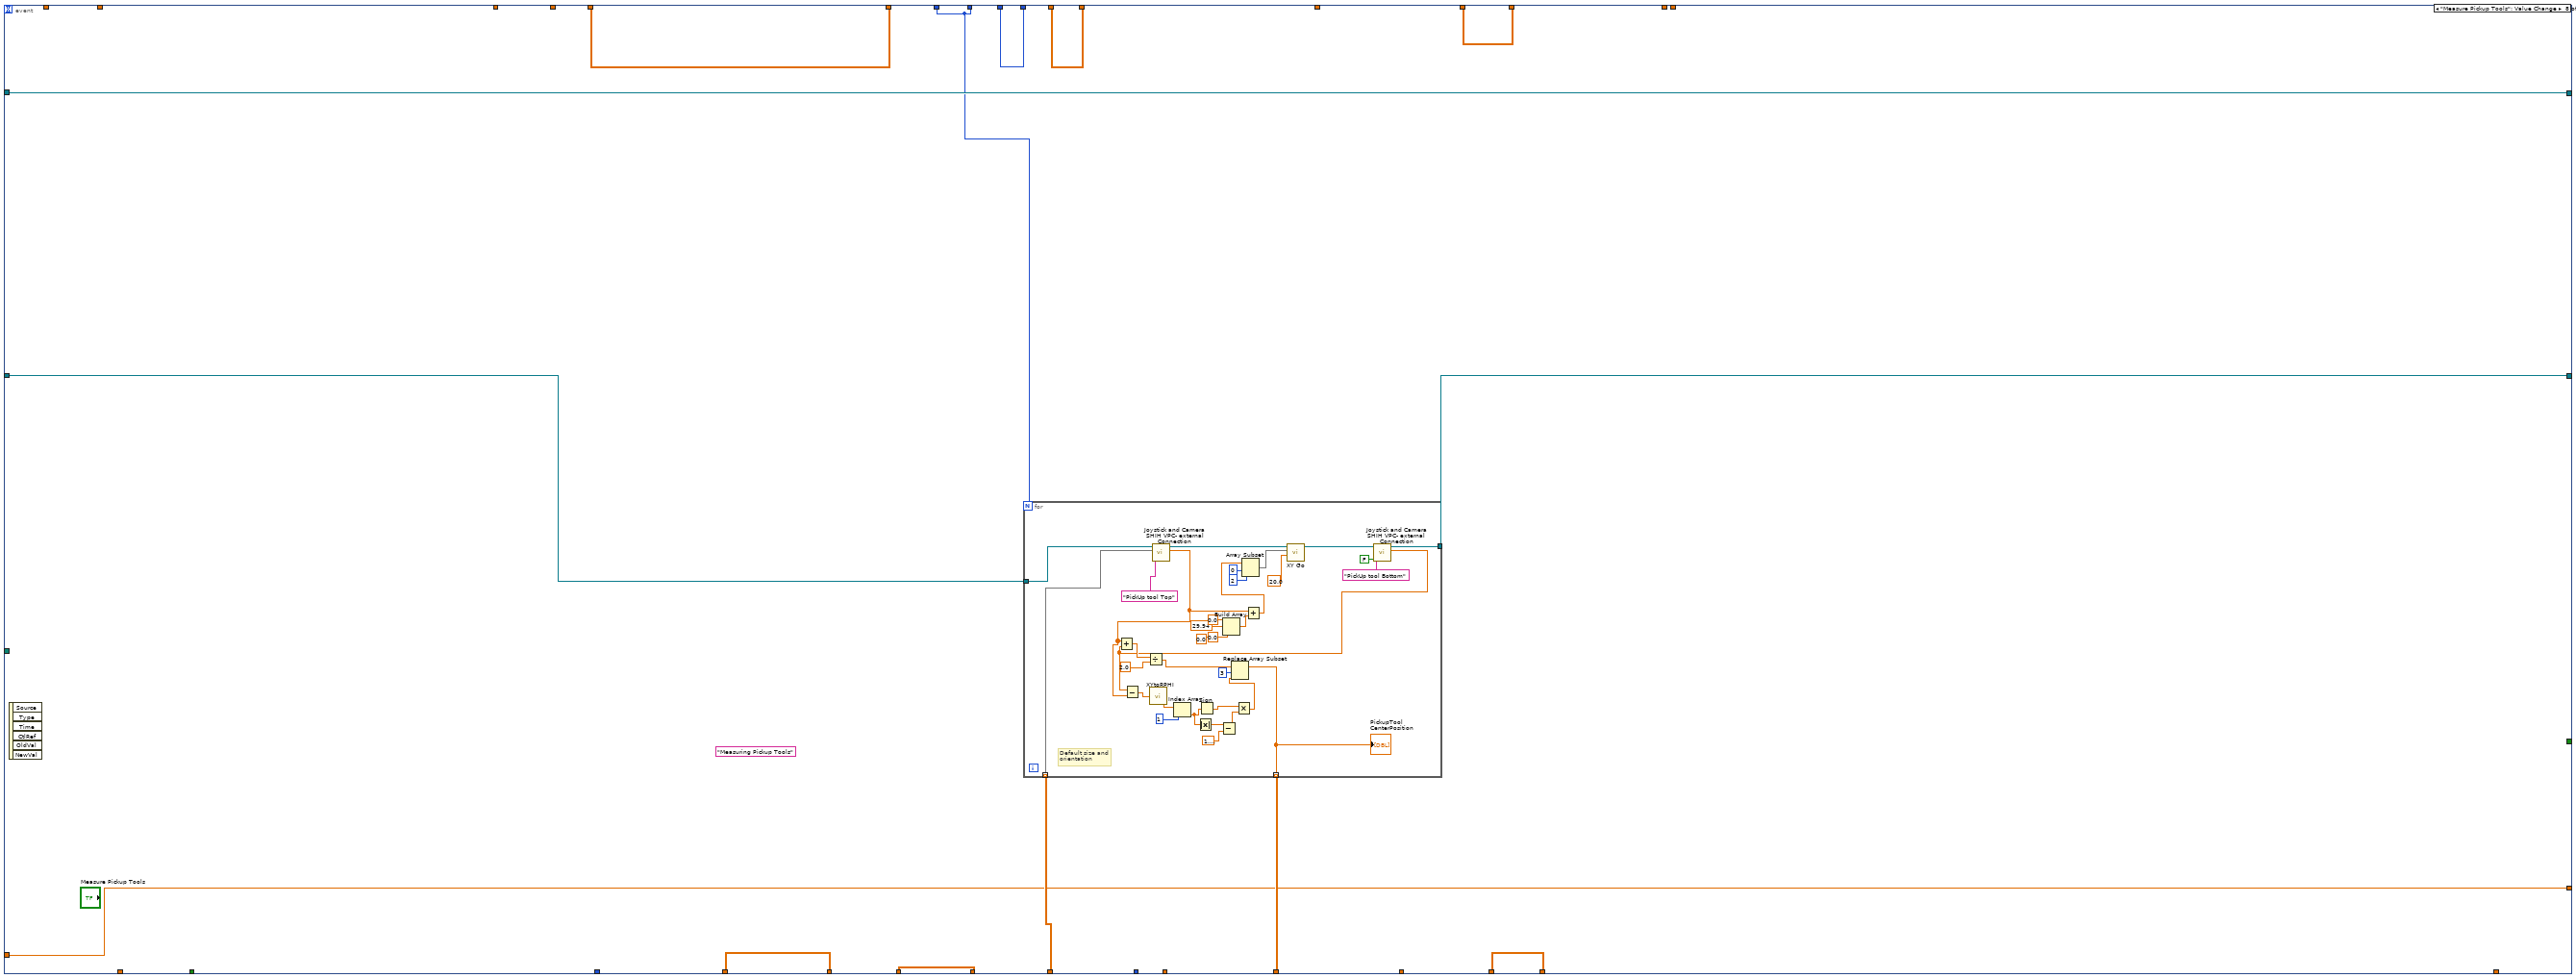
[diagram p16: hidden frame]
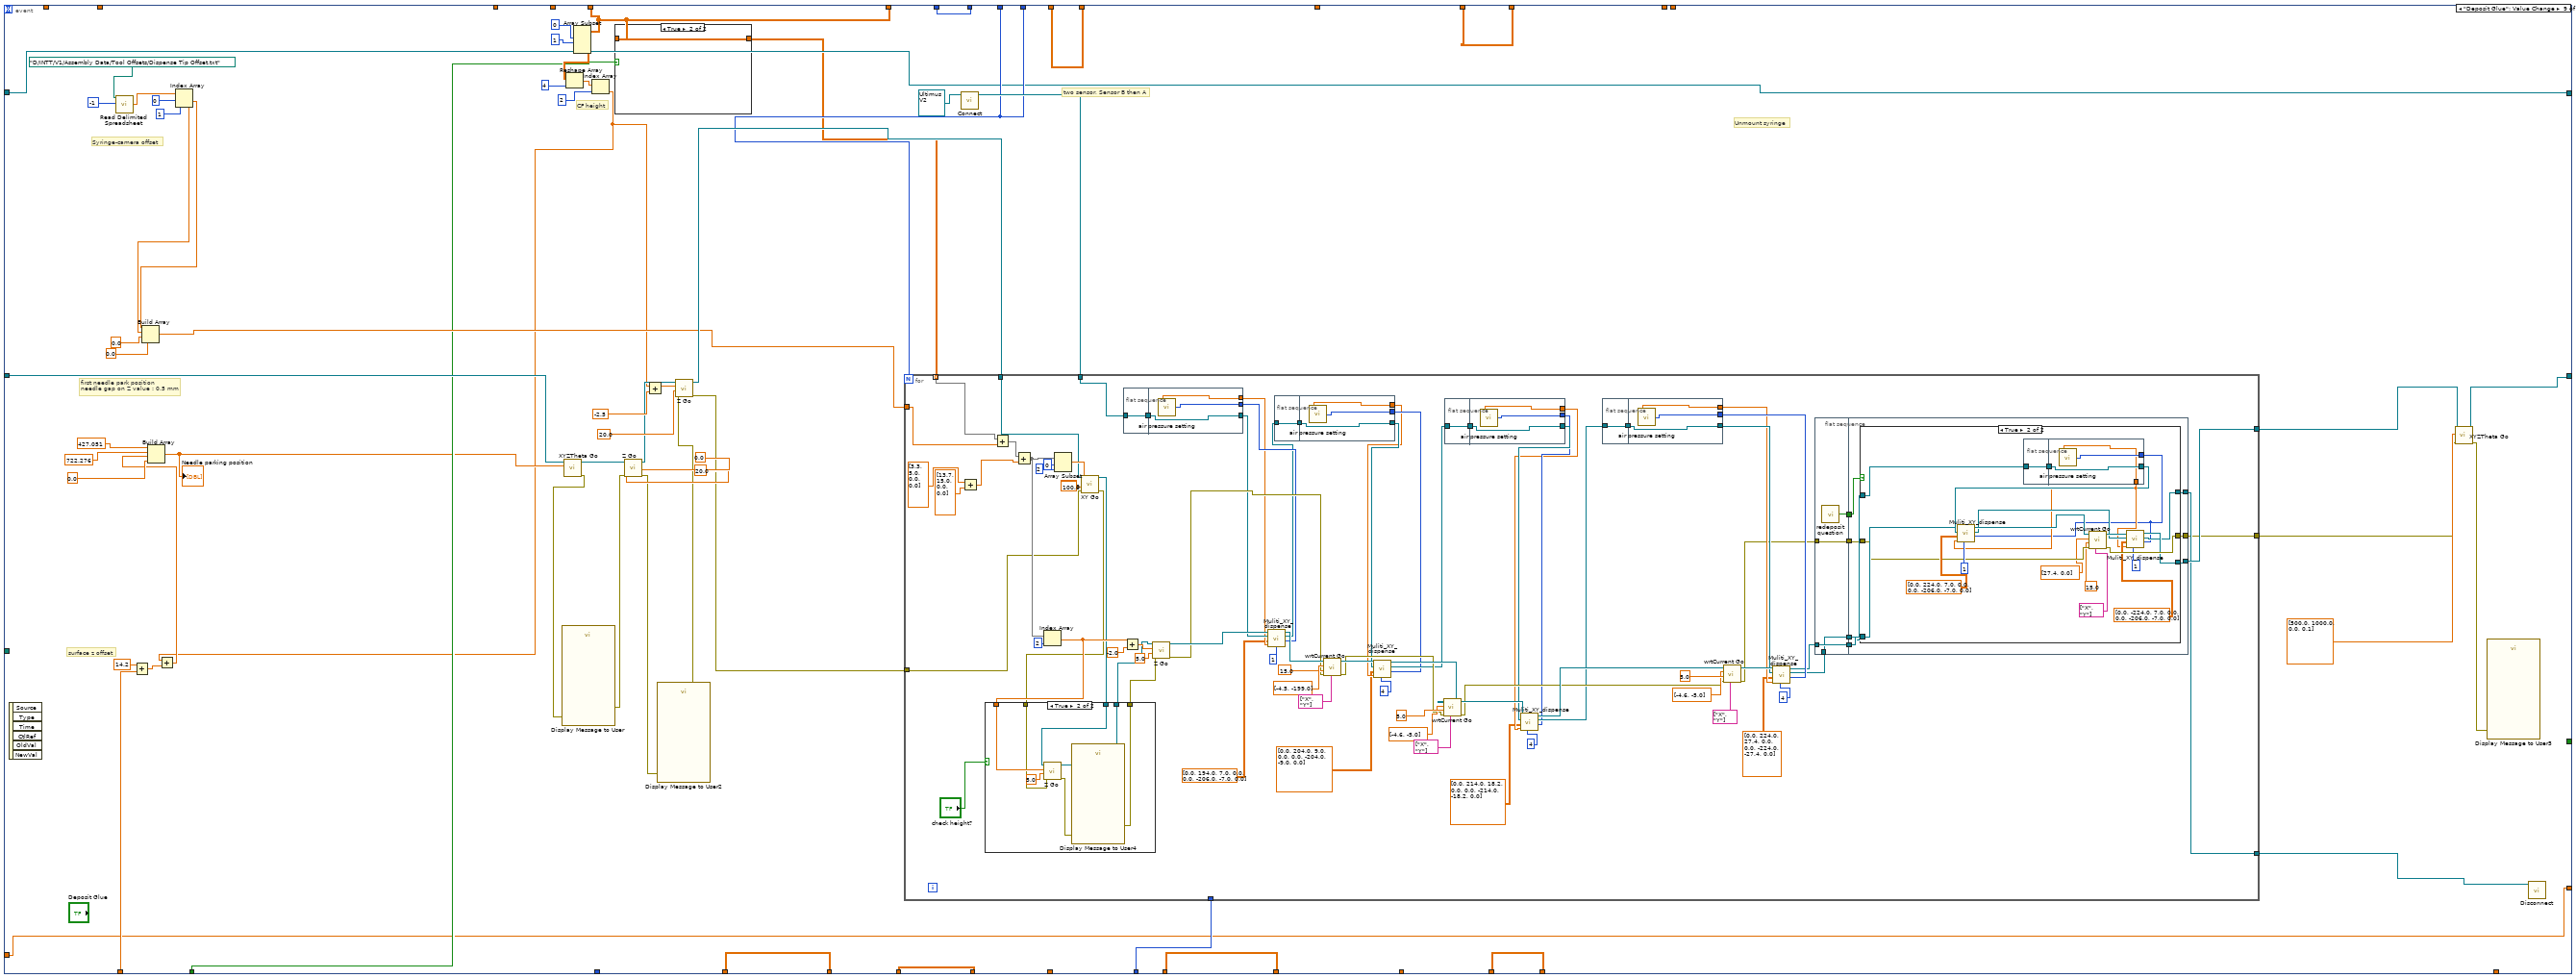
[diagram p17: hidden frame]
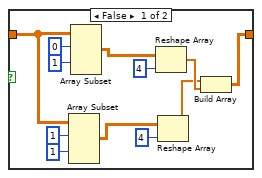
[diagram p18: hidden frame]
diagram:
  w4 = refnum<class "NI-DAQ.lvclass"> refnum  # NI-DAQ.lvclass
  n1 = call "Obtain Control Cluster.vi"("I/O"=FALSE) -> ("Control Out"=w8:T2)  [unwired: 10 in]
  n2 = Unbundle By Name(w8) -> ("Copy of Motion.lvclass"=w6:refnum<class "Motion.lvclass">)
  n3 = call-dynamic "Connect.vi"("NI-DAQ in"=w4) -> ("NI-DAQ out"=w3:refnum<class "NI-DAQ.lvclass">)  [unwired: 9 in, 1 out]
  n4 = while {
    shift-right: [w42] -> w5
    shift-left: w6 -> [w49]
    shift-right: [w22] -> w2
    shift-left: w3 -> [w26]
    shift-right: [w9] -> _
    shift-left: 0.0 -> [w10]
    i -> [w41]
    stop <- w48 stop-if-true
    # "pick&place module"
    # "default module position on stave"
    # "FINAL Pickup tool position"
    # "glue deposit module"
    # "Measured HDI geometry"
    # "module position on tray"
    # "Measured stave top-left"
    # "module on stave"
    n5 = feedback #1() -> (w46:dbl[][])  [unwired: 1 in]
    n6 = feedback #2() -> (w47:dbl[][])  [unwired: 1 in]
    n7 = feedback #3() -> (w23:dbl[][])  [unwired: 1 in]
    n8 = feedback #4() -> (w12:i32)  [unwired: 1 in]
    n9 = feedback #5() -> (w40:i32)  [unwired: 1 in]
    n10 = feedback #6() -> (w35:dbl[][])  [unwired: 1 in]
    n11 = feedback #7() -> (w43:dbl[][])  [unwired: 1 in]
    n12 = call-poly <vilib>:"Read Delimited Spreadsheet.vi"("file path (dialog if empty)"=path "D:/INTT/V1/Assembly Data/ladder assembly/2line_switch.txt" ("file path (dialog if empty) 3"), "format (%.3f)"="%.10f") -> ("all rows"=w14:dbl[][])  [unwired: 8 in, 5 out]
    "file indicator" <- w14
    n13 = feedback #8() -> (w30:dbl[][])  [unwired: 1 in]
    n14 = feedback #9() -> (w11:dbl[][])  [unwired: 1 in]
    "HDI center positions" <- w11
    n15 = event shown="[10] \"Pick and place\": Value Change" {
      selector: _ -> [_ _ _ _ _ _ _ _ _ _ _ _ _ _ _]
      dyn-events: _ -> [_ _ _ _ _ _ _ _ _ _ _ _ _ _ _]
      timeout: 500 -> [_ _ _ _ _ _ _ _ _ _ _ _ _ _ _]
      tunnel: w49 -> [w85 w126 w192 w224 w322 w424 w562 w611 w687 w900 w971 w1149 w1169 w1173 w1196]
      tunnel: [_ _ "Stop" _ _ _ _ _ _ _ _ _ _ _ _] -> w48
      tunnel: [w53 w120 w187 w195 w293 w427 w567 w606 w650 w866 w952 w1155 w1165 w1181 w1195] -> w27
      tunnel: w47 -> [_ w120 w187 _ _ _ w567 w606 w650 w866 w952 w1155 w1165 w1181 w1195]
      tunnel: [w63 w118 w186 w220 w318 w439 w571 w605 w673 w903 w954 w1152 w1164 w1175 w1193] -> w28
      tunnel: w46 -> [_ _ w186 w220 w318 w439 w571 w605 w673 w903 w954 w1152 w1164 w1175 w1193]
      tunnel: w40 -> [_ w113 w189 w225 w323 w442 w566 w602 w676 w905 w948 w1154 w1166 w1179 w1187]
      tunnel: [w68 w117 w184 w227 w325 w444 w568 w604 w675 w901 w939 w1150 w1162 w1177 w1190] -> w45
      tunnel: w11 -> [w68 _ w184 w227 w325 w444 w568 w604 w675 w901 w939 w1150 w1162 w1177 w1190]
      tunnel: [w83 w121 w185 w232 w330 w449 w569 w610 w674 w902 w960 w1151 w1163 w1176 w1191] -> w44
      tunnel: w43 -> [_ w121 w185 w232 w330 w449 w569 _ w674 w902 w960 w1151 w1163 w1176 w1191]
      tunnel: [w85 w125 w190 w221 w319 w440 w560 w609 w677 w892 w961 w1147 w1168 w1173 w1196] -> w42
      tunnel: ["deposit glue module" w113 w189 w225 w323 w442 w566 w602 w676 w905 w948 w1154 w1166 w1179 w1187] -> w39
      tunnel: "Default HDI alignment \nmark position" -> [w66 w124 _ _ _ _ _ _ _ _ _ _ _ _ _]
      tunnel: "Default HDI size" -> [w65 w123 _ _ _ _ _ _ _ _ _ _ _ _ _]
      tunnel: [w72 w122 w188 w226 w324 w443 w565 w607 w672 w904 w959 w1153 w1167 w1180 w1194] -> w36
      tunnel: w35 -> [_ w122 w188 w226 w324 w443 w565 w607 w672 w904 w959 w1153 w1167 w1180 w1194]
      tunnel: "Default Pickup Tool Position" -> [w83 _ _ _ _ _ _ w608 _ _ _ _ _ _ _]
      tunnel: "Uppler / Lower Stave" -> [w69 _ _ w205 w303 w394 _ _ w658 _ w928 _ _ _ _]
      tunnel: "Default Stave upper left mark" -> [w54 _ _ w223 w321 w426 _ _ _ _ _ _ _ _ _]
      tunnel: "Default Stave dimension" -> [w62 _ _ w222 w320 w441 _ _ _ _ _ _ _ _ _]
      tunnel: [w51 w119 w182 w204 w302 w408 w564 w603 w671 w883 w950 w1145 w1159 w1178 w1189] -> w29
      tunnel: w30 -> [w51 w119 w182 _ _ _ w564 w603 w671 w883 w950 w1145 w1159 w1178 w1189]
      tunnel: w26 -> [w61 w115 w180 w203 w301 w435 w559 w600 w666 w881 w957 w1144 w1158 w1185 w1199]
      tunnel: [w61 w115 w180 w203 w301 w435 w557 w600 w666 w881 w956 w1144 w1158 w1172 w1197] -> w22
      tunnel: "HDI vacuum channel" -> [_ _ _ _ _ _ _ _ _ _ w955 _ _ w1182 w1198]
      tunnel: [w64 w116 w181 w219 w317 w438 w570 w601 w667 w882 w953 w1146 w1160 w1174 w1192] -> w24
      tunnel: w23 -> [_ _ w181 w219 w317 w438 w570 w601 w667 w882 w953 w1146 w1160 w1174 w1192]
      tunnel: "Needle Height Compenstation\n(glue gap)" -> [_ _ _ _ _ _ _ _ w660 w874 _ _ _ _ _]
      tunnel: "Uttimus presssure" -> [_ _ _ _ _ _ _ _ w659 _ _ _ _ _ _]
      tunnel: "?" -> [_ _ _ _ _ w425 _ _ _ _ _ _ _ _ _]
      tunnel: [_ _ _ _ _ w423 _ _ _ _ _ _ _ _ _] -> _
      tunnel: "MPT offset" -> [_ _ _ _ _ w409 _ _ _ _ _ _ _ _ _]
      tunnel: w14 -> [_ _ _ _ _ _ _ _ _ _ w951 _ _ _ _]
      tunnel: [1 ("pick &place module") w114 w179 w194 w292 w405 w563 w599 w649 w864 w949 w1143 w1157 w1171 w1188] -> w13
      tunnel: w12 -> [_ w114 w179 w194 w292 w405 w563 w599 w649 w864 w949 w1143 w1157 w1171 w1188]
      tunnel: w11 -> [_ _ _ _ _ _ _ _ _ _ w929 _ _ _ _]
      tunnel: [_ _ _ _ _ w391 _ _ _ _ _ _ _ _ _] -> _
      tunnel: w10 -> [w50 w112 w178 w193 w291 w392 w556 w598 w646 w863 w924 w1142 w1156 w1170 w1186]
      tunnel: [w50 w112 w178 w193 w291 w392 w556 w598 w646 w863 w920 w1142 w1156 w1170 w1186] -> w9
      event "Inititalize": Value Change {
        (unwired) "INITIALIZING ....." ("String")
        (unwired) "ideal delta Y between \n2 fiducial marks"
        (unwired) "ideal delta X between 2 fiducial marks"
        # "center of lower module"
        # "center of upper module"
        n16 = event-data() -> ()  [unwired: 1 in, 6 out]
        n17 = Build Array(17.0 ("element"), 60.9 ("element"), 0.0 ("element"), 0.0 ("element")) -> (w74:dbl[])
        n18 = Build Array(17.0 ("element"), 411.0 ("element"), 0.0 ("element"), 0.0 ("element")) -> (w73:dbl[])
        n19 = case shown="True" w69 {
          tunnel: w74 -> [w94 w97]
          tunnel: w73 -> [w93 w96]
          tunnel: [w92 w95] -> w72
          frame False {
            n20 = Build Array(w93, w94) -> (w92:dbl[][])
          }
          frame True {
            n21 = Build Array(w97, w96) -> (w95:dbl[][])
          }
        }
        "default module position on stave" <- w72
        n22 = Build Array(24.3 ("y"), 231.4 ("y"), 0.0 ("element"), -0.05 ("element")) -> ()  [unwired: 1 out]
        n23 = Build Array(0.0 ("element"), 238.0 ("element"), 0.0 ("element"), 0.0 ("element")) -> (w56:dbl[])
        n24 = Add(x=w54, y=w56) -> (x+y=w55:dbl[])
        n25 = Build Array(w54, w55) -> (w53:dbl[][])
        n26 = for {
          N: 2 -> [_]
          tunnel: w66 -> [w91]
          tunnel: [w91] -> w64 mode=indexing
          tunnel: w65 -> [w90]
          tunnel: [w90] -> w63 mode=indexing
        }
        n27 = Index Array(array=w62, index=3) -> (element=w70:dbl)
        n28 = for {
          tunnel: w72 -> [w105] mode=indexing
          tunnel: w70 -> [w99]
          tunnel: w54 -> [w104]
          tunnel: [w102] -> _ mode=indexing
          (unwired) 0 ("index")
          n29 = Multiply(x=w99, y=-1.0) -> (x*y=w100:dbl)
          n30 = Index Array(array=w105) -> (element=w108:dbl)  [unwired: 1 in]
          n31 = Index Array(array=w105, index=1) -> (element=w107:dbl)
          n32 = call-poly <vilib>:"2D Cartesian Coordinate Rotation.vi"("theta"=w100, "y"=w107, "x"=w108) -> ("y out"=w110:dbl, "x out"=w109:dbl)  [unwired: 6 in, 1 out]
          n33 = Build Array(w109, w110, 0.0 ("element"), 0.0 ("element")) -> (w103:dbl[])
          n34 = Add(x=w103, y=w104) -> (x+y=w102:dbl[])
        }
      }
      event "Measure HDI": Value Change {
        (unwired) "HDI alignment in progress ..." ("String")
        n35 = event-data() -> ()  [unwired: 1 in, 6 out]
        n36 = for {
          N: w114 -> [_]
          tunnel: w123 -> [w140]
          shift-right: [w137] -> w125
          shift-left: w126 -> [w138]
          tunnel: w124 -> [w139]
          tunnel: [w174] -> w116 mode=indexing
          tunnel: [w173] -> w118 mode=indexing
          tunnel: [w127] -> w117 mode=indexing
          (unwired) "ideal delta Y between \n2 fiducial marks"
          (unwired) "ideal delta X between 2 fiducial marks"
          # "1"
          # "3"
          n37 = call "Joystick and Camera SHIH VPC- external Connection.vi"("Motion in"=w138, "XYZTheta"=w139, "Measurement Point"="Measure Top-Left of HDI") -> ("Motion out"=w153:refnum<class "Motion.lvclass">, "Sum"=w130:dbl[])  [unwired: 4 in, 2 out]
          n38 = Add(x=w140, y=w130) -> (x+y=w157:dbl[])
          n39 = Index Array(array=w130, index=0) -> (element=w144:dbl)
          n40 = Array Subset(array=w157, index=0, length=2) -> (w156:dbl[])
          n41 = Replace Array Subset(array=w156, new element=w144, index=0) -> (w154:dbl[])
          n42 = call-dynamic "XY Go.vi"("Speed"=100.0, "XY"=w154, "Motion in"=w153) -> ("Motion out"=w161:refnum<class "Motion.lvclass">)  [unwired: 7 in, 1 out]
          n43 = Build Array(24.3 ("y"), 231.4 ("y"), 0.0 ("element"), -0.05 ("element")) -> ()  [unwired: 1 out]
          n44 = call "Joystick and Camera SHIH VPC- external Connection.vi"("Motion in"=w161, "Measurement Point"="Measure Bottom-Left of HDI", "Inital GO"=FALSE) -> ("Motion out"=w152:refnum<class "Motion.lvclass">, "Sum"=w143:dbl[])  [unwired: 4 in, 2 out]
          n45 = Array Subset(array=w157, index=0, length=2) -> (w167:dbl[])
          n46 = Subtract(x=w143, y=w130) -> (x-y=w151:dbl[])
          n47 = call-dynamic "XY Go.vi"("Speed"=100.0, "XY"=w167, "Motion in"=w152) -> ("Motion out"=w171:refnum<class "Motion.lvclass">)  [unwired: 7 in, 1 out]
          n48 = call "XY_to_Rotation_RPHI.vi"("X-Y"=w151) -> ("r-phi"=w147:dbl[])
          n49 = call "Joystick and Camera SHIH VPC- external Connection.vi"("Motion in"=w171, "Measurement Point"="Measure Bottom-Righ of HDI", "Inital GO"=FALSE) -> ("Motion out"=w137:refnum<class "Motion.lvclass">, "Sum"=w134:dbl[])  [unwired: 4 in, 2 out]
          n50 = Subtract(x=w134, y=w130) -> (x-y=w135:dbl[])
          n51 = Index Array(array=w147, index=1) -> (element=w141:dbl)
          n52 = Multiply(x=w141, y=-1.0) -> (x*y=w132:dbl)
          n53 = Replace Array Subset(array=w135, new element=w132, index=3) -> (w173:dbl[])
          n54 = Replace Array Subset(array=w130, new element=w132, index=3) -> (w174:dbl[])
          n55 = Add(x=w134, y=w130) -> (x+y=w176:dbl[])
          n56 = Divide(x=w176, y=2.0) -> (x/y=w131:dbl[])
          n57 = Replace Array Subset(array=w131, new element=w132, index=3) -> (w128:dbl[])
          n58 = Subtract(x=w128, y=dbl[] [0.4, 0.4, 0.0, 0.0]) -> (x-y=w127:dbl[])
        }
      }
      event "Stop": Value Change {
        n59 = event-data() -> ()  [unwired: 1 in, 6 out]
        n60 = call "XYZTheta Go.vi"("XYZTheta In"=dbl[] [625.0, 625.0, 0.0, 0.01], "Motion in"=w192) -> ("Motion out"=w190:refnum<class "Motion.lvclass">)  [unwired: 7 in, 2 out]
      }
      event "Align Stave": Value Change {
        # "center of lower module"
        # "center of upper module"
        # "Default stave dimension\namong mounting holes"
        # "Measure 2 module positions on stave"
        n61 = event-data() -> ()  [unwired: 1 in, 6 out]
        n62 = Build Array(34.0 ("element"), 470.0 ("element"), 0.0 ("element"), 0.0 ("element")) -> ()  [unwired: 1 out]
        n63 = for {
          N: 1 -> [_]
          tunnel: w222 -> [w239]
          shift-right: [w249] -> w221
          shift-left: w224 -> [w250]
          tunnel: w223 -> [w251]
          tunnel: [w244] -> w197
          tunnel: [w242] -> w207
          (unwired) "ideal delta Y between \n2 fiducial marks"
          (unwired) "ideal delta X between 2 fiducial marks"
          n64 = call "Joystick and Camera SHIH VPC- external Connection.vi"("Motion in"=w250, "XYZTheta"=w251, "Measurement Point"="Measure Top-Left of stave") -> ("Motion out"=w233:refnum<class "Motion.lvclass">, "Sum"=w235:dbl[])  [unwired: 4 in, 2 out]
          n65 = Replace Array Subset(array=w239, new element=0.0 ("new element/subarray"), index=0) -> (w236:dbl[])
          n66 = Add(x=w235, y=w236) -> (x+y=w234:dbl[])
          n67 = call "Joystick and Camera SHIH VPC- external Connection.vi"("Motion in"=w233, "XYZTheta"=w234, "Measurement Point"="Measure Bottom-Left of stave", "Inital GO"=TRUE) -> ("Motion out"=w241:refnum<class "Motion.lvclass">, "Sum"=w254:dbl[])  [unwired: 3 in, 2 out]
          n68 = Build Array(24.3 ("y"), 231.4 ("y"), 0.0 ("element"), -0.05 ("element")) -> ()  [unwired: 1 out]
          n69 = Add(x=w239, y=w235) -> (x+y=w240:dbl[])
          n70 = Subtract(x=w254, y=w235) -> (x-y=w260:dbl[])
          n71 = call "XY_to_Rotation_RPHI.vi"("X-Y"=w260) -> ("r-phi"=w256:dbl[])
          n72 = Index Array(array=w256, index=1) -> (element=w252:dbl)
          n73 = call "Joystick and Camera SHIH VPC- external Connection.vi"("Motion in"=w241, "XYZTheta"=w240, "Measurement Point"="Measure Bottom-Righ of stave", "Inital GO"=TRUE) -> ("Motion out"=w249:refnum<class "Motion.lvclass">, "Sum"=w246:dbl[])  [unwired: 3 in, 2 out]
          n74 = Subtract(x=w246, y=w235) -> (x-y=w247:dbl[])
          n75 = Multiply(x=w252, y=-1.0) -> (x*y=w242:dbl)
          n76 = Replace Array Subset(array=w247, new element=w242, index=3) -> (→"measured stave size":dbl[])
          n77 = Replace Array Subset(array=w235, new element=w242, index=3) -> (w244:dbl[])
          n78 = Add(x=w246, y=w235) -> (x+y=w268:dbl[])
          n79 = Divide(x=w268, y=2.0) -> (x/y=→"Center of module on stave":dbl[])
        }
        n80 = Build Array(0.0 ("element"), 238.0 ("element"), 0.0 ("element"), 0.0 ("element")) -> (w198:dbl[])
        n81 = Add(x=w197, y=w198) -> (x+y=w196:dbl[])
        n82 = Build Array(w197, w196) -> (w195:dbl[][])
        n83 = Build Array(17.0 ("element"), 411.0 ("element"), 0.0 ("element"), 0.0 ("element")) -> (w209:dbl[])
        n84 = Build Array(17.0 ("element"), 60.9 ("element"), 0.0 ("element"), 0.0 ("element")) -> (w210:dbl[])
        n85 = case shown="True" w205 {
          tunnel: w210 -> [w287 w290]
          tunnel: w209 -> [w286 w289]
          tunnel: [w285 w288] -> w208
          frame False {
            n86 = Build Array(w286, w287) -> (w285:dbl[][])
          }
          frame True {
            n87 = Build Array(w290, w289) -> (w288:dbl[][])
          }
        }
        n88 = for {
          tunnel: w208 -> [w278] mode=indexing
          tunnel: w207 -> [w273]
          tunnel: w197 -> [w277]
          tunnel: [w275] -> w204 mode=indexing
          n89 = Multiply(x=w273, y=-1.0) -> (x*y=w272:dbl)
          n90 = Index Array(array=w278, index=0) -> (element=w281:dbl)
          n91 = Index Array(array=w278, index=1) -> (element=w280:dbl)
          n92 = call-poly <vilib>:"2D Cartesian Coordinate Rotation.vi"("theta"=w272, "y"=w280, "x"=w281) -> ("y out"=w283:dbl, "x out"=w282:dbl)  [unwired: 6 in, 1 out]
          n93 = Build Array(w282, w283, 0.0 ("element"), 0.0 ("element")) -> (w276:dbl[])
          n94 = Add(x=w276, y=w277) -> (x+y=w275:dbl[])
        }
      }
      event "Align Stave in detail": Value Change {
        # "center of lower module"
        # "center of upper module"
        # "Default stave dimension\namong mounting holes"
        # "Measure 2 module positions on stave"
        n95 = event-data() -> ()  [unwired: 1 in, 6 out]
        n96 = Build Array(34.0 ("element"), 470.0 ("element"), 0.0 ("element"), 0.0 ("element")) -> ()  [unwired: 1 out]
        n97 = for {
          N: 1 -> [_]
          tunnel: w320 -> [w337]
          shift-right: [w347] -> w319
          shift-left: w322 -> [w348]
          tunnel: w321 -> [w349]
          tunnel: [w342] -> w295
          tunnel: [w340] -> w305
          (unwired) "ideal delta Y between \n2 fiducial marks"
          (unwired) "ideal delta X between 2 fiducial marks"
          n98 = call "Joystick and Camera SHIH V5- external Connection.vi"("Motion in"=w348, "XYZTheta"=w349, "Measurement Point"="Measure Top-Left of stave") -> ("final out"=w333:dbl[], "Motion out"=w331:refnum<class "Motion.lvclass">)  [unwired: 5 in, 1 out]
          n99 = Replace Array Subset(array=w337, new element=0.0 ("new element/subarray"), index=0) -> (w334:dbl[])
          n100 = Add(x=w333, y=w334) -> (x+y=w332:dbl[])
          n101 = call "Joystick and Camera SHIH V5- external Connection.vi"("Motion in"=w331, "XYZTheta"=w332, "Measurement Point"="Measure Bottom-Left of stave", "Inital GO"=TRUE) -> ("final out"=w352:dbl[], "Motion out"=w339:refnum<class "Motion.lvclass">)  [unwired: 4 in, 1 out]
          n102 = Build Array(24.3 ("y"), 231.4 ("y"), 0.0 ("element"), -0.05 ("element")) -> ()  [unwired: 1 out]
          n103 = Add(x=w337, y=w333) -> (x+y=w338:dbl[])
          n104 = Subtract(x=w352, y=w333) -> (x-y=w358:dbl[])
          n105 = call "XY_to_Rotation_RPHI.vi"("X-Y"=w358) -> ("r-phi"=w354:dbl[])
          n106 = Index Array(array=w354, index=1) -> (element=w350:dbl)
          n107 = call "Joystick and Camera SHIH V5- external Connection.vi"("Motion in"=w339, "XYZTheta"=w338, "Measurement Point"="Measure Bottom-Righ of stave", "Inital GO"=TRUE) -> ("final out"=w344:dbl[], "Motion out"=w347:refnum<class "Motion.lvclass">)  [unwired: 4 in, 1 out]
          n108 = Subtract(x=w344, y=w333) -> (x-y=w345:dbl[])
          n109 = Multiply(x=w350, y=-1.0) -> (x*y=w340:dbl)
          n110 = Replace Array Subset(array=w345, new element=w340, index=3) -> (→"FROM Detail !! measured stave size":dbl[])
          n111 = Replace Array Subset(array=w333, new element=w340, index=3) -> (w342:dbl[])
          n112 = Add(x=w344, y=w333) -> (x+y=w366:dbl[])
          n113 = Divide(x=w366, y=2.0) -> (x/y=→"FROM Detail !!! Center of module on stave":dbl[])
        }
        n114 = Build Array(0.0 ("element"), 238.0 ("element"), 0.0 ("element"), 0.0 ("element")) -> (w296:dbl[])
        n115 = Add(x=w295, y=w296) -> (x+y=w294:dbl[])
        n116 = Build Array(w295, w294) -> (w293:dbl[][])
        n117 = Build Array(17.0 ("element"), 411.0 ("element"), 0.0 ("element"), 0.0 ("element")) -> (w307:dbl[])
        n118 = Build Array(17.0 ("element"), 60.9 ("element"), 0.0 ("element"), 0.0 ("element")) -> (w308:dbl[])
        n119 = case shown="True" w303 {
          tunnel: w308 -> [w385 w388]
          tunnel: w307 -> [w384 w387]
          tunnel: [w383 w386] -> w306
          frame False {
            n120 = Build Array(w384, w385) -> (w383:dbl[][])
          }
          frame True {
            n121 = Build Array(w388, w387) -> (w386:dbl[][])
          }
        }
        n122 = for {
          tunnel: w306 -> [w376] mode=indexing
          tunnel: w305 -> [w371]
          tunnel: w295 -> [w375]
          tunnel: [w373] -> w302 mode=indexing
          n123 = Multiply(x=w371, y=-1.0) -> (x*y=w370:dbl)
          n124 = Index Array(array=w376, index=0) -> (element=w379:dbl)
          n125 = Index Array(array=w376, index=1) -> (element=w378:dbl)
          n126 = call-poly <vilib>:"2D Cartesian Coordinate Rotation.vi"("theta"=w370, "y"=w378, "x"=w379) -> ("y out"=w381:dbl, "x out"=w380:dbl)  [unwired: 6 in, 1 out]
          n127 = Build Array(w380, w381, 0.0 ("element"), 0.0 ("element")) -> (w374:dbl[])
          n128 = Add(x=w374, y=w375) -> (x+y=w373:dbl[])
        }
      }
      event "Bless from OGP": Value Change {
        # "stave center position on gantry"
        # "center of upper module"
        # "center of lower module"
        # "center of upper module"
        # "NL line with correct rotation"
        # "Default stave dimension\namong mounting holes"
        # "Measure 2 module positions on stave"
        n129 = event-data() -> ()  [unwired: 1 in, 6 out]
        n130 = Build Array(34.0 ("element"), 470.0 ("element"), 0.0 ("element"), 0.0 ("element")) -> ()  [unwired: 1 out]
        n131 = for {
          N: 1 -> [_]
          tunnel: w441 -> [_]
          shift-right: [w501] -> w440
          shift-left: w424 -> [w514]
          tunnel: w426 -> [_]
          tunnel: [w493] -> w429
          tunnel: [w496] -> w437
          tunnel: w425 -> [w503]
          tunnel: [w479] -> w412
          (unwired) FALSE ("Inital GO")
          (unwired) "ideal delta Y between \n2 fiducial marks"
          (unwired) "ideal delta X between 2 fiducial marks"
          # "after NL"
          # "after SL"
          # "NL line"
          # "rotation"
          n132 = call "Joystick and Camera SHIH VPC- external Connection.vi"("Motion in"=w514, "XYZTheta"=dbl[] [576.333, 663.131, 66.662912, 0.010000094994154989] ("N chip"), "Measurement Point"="north chip", "Inital GO"=TRUE) -> ("Motion out"=w511:refnum<class "Motion.lvclass">, "Sum"=w491:dbl[])  [unwired: 3 in, 2 out]
          "N chip" <- w491
          n133 = call "Joystick and Camera SHIH VPC- external Connection.vi"("Motion in"=w511, "XYZTheta"=dbl[] [578.791, 1154.64, 66.662912, 0.010000670236950445] ("S chip"), "Measurement Point"="south chip", "Inital GO"=TRUE) -> ("Motion out"=w510:refnum<class "Motion.lvclass">, "Sum"=w492:dbl[])  [unwired: 3 in, 2 out]
          "S chip" <- w492
          n134 = Subtract(x=w492, y=w491) -> (x-y=w490:dbl[])
          n135 = Index Array(array=w490, index #1=0 ("index"), index #2=1 ("index")) -> (element #1=w487:dbl, element #2=w486:dbl)
          n136 = Square(x=w487) -> (x^2=w484:dbl)
          n137 = Square(x=w486) -> (x^2=w485:dbl)
          n138 = Add(x=w484, y=w485) -> (x+y=w483:dbl)
          n139 = call "Joystick and Camera SHIH VPC- external Connection.vi"("Motion in"=w510, "Measurement Point"="height of stave", "Inital GO"=FALSE) -> ("Motion out"=w501:refnum<class "Motion.lvclass">, "Sum"=w502:dbl[])  [unwired: 4 in, 2 out]
          n140 = call "O to G peek.vi"("height"=w502, "south chip"=w492, "north chip"=w491, "Input file"=w503) -> ("OGP length"=→"chip distance by OGP":dbl, "output BR"=w505:dbl[], "output BL"=w504:dbl[], "output TL"=w498:dbl[])  [unwired: 4 in]
          "after NL" <- w498
          "after SR" <- w505
          "after SL" <- w504
          n141 = Square Root(x=w483) -> (sqrt(x)=→"chip distance by gantry":dbl)
          n142 = Subtract(x=w505, y=w498) -> (x-y=w516:dbl[])
          n143 = Build Array(24.3 ("y"), 231.4 ("y"), 0.0 ("element"), -0.05 ("element")) -> ()  [unwired: 1 out]
          n144 = Subtract(x=w504, y=w498) -> (x-y=w522:dbl[])
          n145 = call "XY_to_Rotation_RPHI.vi"("X-Y"=w522) -> ("r-phi"=w521:dbl[])
          n146 = Index Array(array=w521, index=1) -> (element=w518:dbl)
          n147 = Multiply(x=w518, y=-1.0) -> (x*y=w496:dbl)
          n148 = Replace Array Subset(array=w516, new element=w496, index=3) -> (→"bless from OGP !! measured stave size":dbl[])
          n149 = Replace Array Subset(array=w498, new element=w496, index=3) -> (w494:dbl[])
          n150 = Add(x=w505, y=w498) -> (x+y=w528:dbl[])
          n151 = Divide(x=w528, y=2.0) -> (x/y=w480:dbl[])
          n152 = Add(x=w494, y=dbl[] [0.0, 10.0, 0.0, 0.0]) -> (x+y=w493:dbl[])
          n153 = Replace Array Subset(array=w480, new element=w496, index=3) -> (w479:dbl[])
          "bless from OGP !!! Center of  stave" <- w479
        }
        n154 = Build Array(0.0 ("element"), 238.0 ("element"), 0.0 ("element"), 0.0 ("element")) -> (w430:dbl[])
        n155 = Add(x=w429, y=w430) -> (x+y=w428:dbl[])
        n156 = Build Array(w429, w428) -> (w427:dbl[][])
        n157 = Build Array(0.0 ("element"), 116.65 ("element"), 0.0 ("element"), 0.0 ("element")) -> (w413:dbl[])
        n158 = Build Array(0.0 ("element"), -116.65 ("element"), 0.0 ("element"), 0.0 ("element")) -> (w414:dbl[])
        n159 = Build Array(0.0 ("element"), 116.65 ("element"), 0.0 ("element"), 0.0 ("element")) -> (w395:dbl[])
        n160 = Build Array(0.0 ("element"), -116.65 ("element"), 0.0 ("element"), 0.0 ("element")) -> (w396:dbl[])
        n161 = case shown="False" w394 {
          tunnel: w414 -> [w475 w478]
          tunnel: w413 -> [w474 w477]
          tunnel: [w473 w476] -> w411
          frame False {
            n162 = Build Array(w474, w475) -> (w473:dbl[][])
          }
          frame True {
            n163 = Build Array(w478, w477) -> (w476:dbl[][])
          }
        }
        n164 = case shown="False" w394 {
          tunnel: w396 -> [w452 w455]
          tunnel: w395 -> [w451 w454]
          tunnel: [w450 w453] -> w393
          frame False {
            n165 = Build Array(w451, w452) -> (w450:dbl[][])
          }
          frame True {
            n166 = Build Array(w455, w454) -> (w453:dbl[][])
          }
        }
        n167 = for {
          tunnel: w411 -> [w549] mode=indexing
          tunnel: w437 -> [w546]
          tunnel: [w548] -> w423 mode=indexing
          tunnel: w412 -> [w531]
          tunnel: [w543] -> w410 mode=indexing
          tunnel: w393 -> [w534] mode=indexing
          tunnel: [w530] -> w391 mode=indexing
          n168 = Multiply(x=w546, y=-1.0) -> (x*y=w533:dbl)
          n169 = Index Array(array=w549, index=0) -> (element=w552:dbl)
          n170 = Index Array(array=w549, index=1) -> (element=w551:dbl)
          n171 = Index Array(array=w534, index=0) -> (element=w539:dbl)
          n172 = Index Array(array=w534, index=1) -> (element=w538:dbl)
          n173 = call-poly <vilib>:"2D Cartesian Coordinate Rotation.vi"("theta"=w533, "y"=w551, "x"=w552) -> ("y out"=w554:dbl, "x out"=w553:dbl)  [unwired: 6 in, 1 out]
          n174 = call-poly <vilib>:"2D Cartesian Coordinate Rotation.vi"("theta"=w533, "y"=w538, "x"=w539) -> ("y out"=w541:dbl, "x out"=w540:dbl)  [unwired: 6 in, 1 out]
          n175 = Build Array(w553, w554, 0.0 ("element"), 0.0 ("element")) -> (w543:dbl[])
          n176 = Build Array(w540, w541, 0.0 ("element"), 0.0 ("element")) -> (w532:dbl[])
          n177 = Add(x=w532, y=w531) -> (x+y=w530:dbl[])
          n178 = Add(x=w543, y=w531) -> (x+y=w548:dbl[])
        }
        "CT HPoS" <- w410
        "HDI center positions" <- w391
        n179 = Add(x=w423, y=w409) -> (x+y=w408:dbl[][])
        n180 = call-poly <vilib>:"Write Delimited Spreadsheet.vi"("file path (dialog if empty)"=path "D:/INTT/V1/Assembly Data/ladder assembly/2line_switch.txt", "format (%.3f)"="%.10f", "2D data"=w408) -> ()  [unwired: 11 in, 2 out]
        n181 = disable-structure shown="Disabled" {
          disable-tunnel: w394 -> [w456 _]
          frame Disabled {
            # "center of lower module"
            # "center of upper module"
            n182 = Build Array(17.0 ("element"), 60.9 ("element"), 0.0 ("element"), 0.0 ("element")) -> (w458:dbl[])
            n183 = Build Array(17.0 ("element"), 411.0 ("element"), 0.0 ("element"), 0.0 ("element")) -> (w457:dbl[])
            n184 = case shown="True" w456 {
              tunnel: w458 -> [w469 w472]
              tunnel: w457 -> [w468 w471]
              tunnel: [w467 w470] -> _
              frame False {
                n185 = Build Array(w468, w469) -> (w467:dbl[][])
              }
              frame True {
                n186 = Build Array(w472, w471) -> (w470:dbl[][])
              }
            }
          }
          frame Enabled {
          }
        }
        n187 = call-poly <vilib>:"Write Delimited Spreadsheet.vi"("file path (dialog if empty)"=path "D:/INTT/V1/Assembly Data/ladder assembly/stave_HDI_center.txt", "format (%.3f)"="%.8f", "2D data"=w391) -> ()  [unwired: 11 in, 2 out]
      }
      event "txt switch": Value Change {
        n188 = event-data() -> ()  [unwired: 1 in, 6 out]
        n189 = flat-sequence {
          tunnel: [w578] -> w572
          tunnel: w562 -> [w574]
          tunnel: [w574] -> w561
          tunnel: w559 -> [w573]
          tunnel: [w573] -> w558
          tunnel: w572 -> [w596]
          tunnel: [w594] -> w560
          tunnel: w561 -> [w594]
          tunnel: [w593] -> w557
          tunnel: w558 -> [w593]
          frame #0 {
            n190 = call-poly <vilib>:"Read Delimited Spreadsheet.vi"("file path (dialog if empty)"=path "D:/INTT/V1/Assembly Data/ladder assembly/2line_switch.txt" ("file path (dialog if empty) 3"), "format (%.3f)"="%.10f") -> ("all rows"=w579:dbl[][])  [unwired: 8 in, 5 out]
            n191 = Array Subset(array=w579, index (row)=0 ("index"), length (row)=1 ("length"), index (col)=0 ("index"), length (col)=4 ("length")) -> (w589:dbl[][])
            n192 = Reshape Array(w589, 4 ("dimension size")) -> (w576:dbl[])
            n193 = Array Subset(array=w579, index (row)=1 ("index"), length (row)=1 ("length"), index (col)=0 ("index"), length (col)=4 ("length")) -> (w583:dbl[][])
            n194 = Reshape Array(w583, 4 ("dimension size")) -> (w577:dbl[])
            n195 = Build Array(w577, w576) -> (w578:dbl[][])
          }
          frame #1 {
            n196 = call-poly <vilib>:"Write Delimited Spreadsheet.vi"("file path (dialog if empty)"=path "D:/INTT/V1/Assembly Data/ladder assembly/2line_switch.txt" ("file path (dialog if empty) 4"), "format (%.3f)"="%.10f", "2D data"=w596) -> ()  [unwired: 11 in, 2 out]
          }
        }
      }
      event "Measure Pickup Tools": Value Change {
        (unwired) "Measuring Pickup Tools" ("String")
        n197 = event-data() -> ()  [unwired: 1 in, 6 out]
        n198 = for {
          N: w599 -> [_]
          tunnel: [w635] -> w610 mode=indexing
          tunnel: w611 -> [w639]
          tunnel: [w621] -> w609
          tunnel: w608 -> [w620] mode=indexing
          # "Default size and\norientation"
          n199 = call "Joystick and Camera SHIH VPC- external Connection.vi"("Motion in"=w639, "XYZTheta"=w620, "Measurement Point"="PickUp tool Top") -> ("Motion out"=w615:refnum<class "Motion.lvclass">, "Sum"=w638:dbl[])  [unwired: 4 in, 2 out]
          n200 = Build Array(0.0 ("element"), 29.94 ("element"), 0.0 ("element"), 0.0 ("element")) -> (w626:dbl[])
          n201 = Add(x=w638, y=w626) -> (x+y=w612:dbl[])
          n202 = Array Subset(array=w612, index=0, length=2) -> (w613:dbl[])
          n203 = call-dynamic "XY Go.vi"("Speed"=20.0, "XY"=w613, "Motion in"=w615) -> ("Motion out"=w614:refnum<class "Motion.lvclass">)  [unwired: 7 in, 1 out]
          n204 = call "Joystick and Camera SHIH VPC- external Connection.vi"("Motion in"=w614, "Measurement Point"="PickUp tool Bottom", "Inital GO"=FALSE) -> ("Motion out"=w621:refnum<class "Motion.lvclass">, "Sum"=w637:dbl[])  [unwired: 4 in, 2 out]
          n205 = Add(x=w638, y=w637) -> (x+y=w644:dbl[])
          n206 = Subtract(x=w637, y=w638) -> (x-y=w636:dbl[])
          n207 = Divide(x=w644, y=2.0) -> (x/y=w641:dbl[])
          n208 = call "XYtoRPHI.vi"("X-Y"=w636) -> ("r-phi"=w642:dbl[])
          n209 = Index Array(array=w642, index=1) -> (element=w630:dbl)
          n210 = Absolute Value(x=w630) -> (abs(x)=w633:dbl)
          n211 = Sign(1:w630) -> (0:w631:dbl)
          n212 = Subtract(x=w633, y=1.5707963267948966) -> (x-y=w632:dbl)
          n213 = Multiply(x=w631, y=w632) -> (x*y=w629:dbl)
          n214 = Replace Array Subset(array=w641, new element=w629, index=3) -> (w635:dbl[])
          "PickupTool \nCenterPosition" <- w635
        }
      }
      event "Deposit Glue": Value Change {
        # "CF height"
        # "surface z offset"
        # "two sensor, Sensor B then A"
        # "Unmount syringe"
        # "first needle park position\nneedle gap on Z value : 0.5 mm"
        # "Syringe-camera offset"
        n215 = event-data() -> ()  [unwired: 1 in, 6 out]
        n216 = call-poly <vilib>:"Read Delimited Spreadsheet.vi"("file path (dialog if empty)"=path "D:/INTT/V1/Assembly Data/Tool Offsets/Dispense Tip Offset.txt", "number of rows (all:-1)"=-1) -> ("first row"=w702:dbl[])  [unwired: 8 in, 5 out]
        n217 = Add(x=14.2 ("element"), y=w660) -> (x+y=w654:dbl)
        n218 = Index Array(array=w702, index #1=0 ("index"), index #2=1 ("index")) -> (element #1=w647:dbl, element #2=w696:dbl)
        n219 = Build Array(w647, w696, 0.0 ("element"), 0.0 ("element")) -> (w682:dbl[])
        n220 = Array Subset(array=w650, index (row)=0, length (row)=1 ("length")) -> (w662:dbl[][])  [unwired: 2 in]
        n221 = Reshape Array(w662, 4 ("dimension size")) -> (w656:dbl[])
        n222 = Index Array(array=w656, index=2) -> (element=w651:dbl)
        n223 = Add(x=w651, y=w654) -> (x+y=w653:dbl)
        n224 = Build Array(427.051, 722.276, w653, 0.0 ("element")) -> (w652:dbl[])
        "Needle parking position" <- w652
        n225 = call "XYZTheta Go.vi"("XYZTheta In"=w652, "Motion in"=w687) -> ("error out"=w695:errorcluster, "Motion out"=w686:refnum<class "Motion.lvclass">)  [unwired: 7 in, 1 out]
        n226 = call "Display Message to User"("error in (no error)"=w695) -> ("error out"=w688:errorcluster)  [unwired: 9 in, 1 out]
        n227 = case shown="True" w658 {
          tunnel: w650 -> [w710 w719]
          tunnel: [w707 w719] -> w657
          frame False {
            n228 = Array Subset(array=w710, index (row)=1 ("index"), length (row)=1 ("length")) -> (w711:dbl[][])  [unwired: 2 in]
            n229 = Array Subset(array=w710, index (row)=0 ("index"), length (row)=1 ("length")) -> (w714:dbl[][])  [unwired: 2 in]
            n230 = Reshape Array(w714, 4 ("dimension size")) -> (w709:dbl[])
            n231 = Reshape Array(w711, 4 ("dimension size")) -> (w708:dbl[])
            n232 = Build Array(w708, w709) -> (w707:dbl[][])
          }
          frame True {
          }
        }
        n233 = call-dynamic "Z Go.vi"("error in (no error)"=w688, "Speed"=20.0, "Position"=0.0, "Motion in"=w686) -> ("error out"=w685:errorcluster, "Motion out"=w691:refnum<class "Motion.lvclass">)  [unwired: 6 in]
        n234 = Add(x=w651, y=-2.5) -> (x+y=w692:dbl)
        n235 = call "Display Message to User2"("error in (no error)"=w685) -> ("error out"=w684:errorcluster)  [unwired: 9 in, 1 out]
        n236 = call-dynamic "Z Go.vi"("error in (no error)"=w684, "Speed"=20.0, "Position"=w692, "Motion in"=w691) -> ("error out"=w661:errorcluster, "Motion out"=w683:refnum<class "Motion.lvclass">)  [unwired: 6 in]
        n237 = call-dynamic "Connect.vi"("Ultimus V in"=refnum<class "Ultimus V2.lvclass"> refnum ("Ultimus V2.lvclass")) -> ("Ultimus V out"=w681:refnum<class "Ultimus V2.lvclass">)  [unwired: 9 in, 1 out]
        n238 = for {
          N: w676 -> [_]
          tunnel: w683 -> [w766]
          tunnel: w681 -> [w756]
          tunnel: w682 -> [w767]
          tunnel: w657 -> [w768] mode=indexing
          tunnel: [w725] -> w669
          tunnel: [w724] -> w668
          tunnel: w661 -> [w763]
          tunnel: w659 -> [_]
          tunnel: [w720] -> w648
          (unwired) 100.0 ("Speed")
          n239 = Add(x=dbl[] [3.3, 5.0, 0.0, 0.0] ("y"), y=dbl[] [13.7, 15.0, 0.0, 0.0]) -> (x+y=w734:dbl[])
          n240 = Add(x=w768, y=w767) -> (x+y=w791:dbl[])
          n241 = Add(x=w791, y=w734) -> (x+y=w792:dbl[])
          n242 = Index Array(array=w792, index=2) -> (element=w761:dbl)
          n243 = Array Subset(array=w792, index=0, length=2) -> (w773:dbl[])
          n244 = call-dynamic "XY Go.vi"("error in (no error)"=w763, "Speed"=100.0, "XY"=w773, "Motion in"=w766) -> ("error out"=w759:errorcluster, "Motion out"=w760:refnum<class "Motion.lvclass">)  [unwired: 6 in]
          n245 = case shown="True" "check height?" {
            tunnel: w761 -> [_ w861]
            tunnel: w760 -> [w854 w860]
            tunnel: w759 -> [w855 w859]
            tunnel: [w855 w857] -> w758
            tunnel: [w854 w856] -> w757
            frame False {
            }
            frame True {
              n246 = call-dynamic "Z Go.vi"("error in (no error)"=w859, "Speed"=5.0, "Position"=w861, "Motion in"=w860) -> ("error out"=w858:errorcluster, "Motion out"=w856:refnum<class "Motion.lvclass">)  [unwired: 6 in]
              n247 = call "Display Message to User4"("error in (no error)"=w858) -> ("error out"=w857:errorcluster)  [unwired: 9 in, 1 out]
            }
          }
          n248 = flat-sequence {
            tunnel: w756 -> [w850]
            tunnel: [w850] -> w755
            tunnel: w755 -> [w853]
            tunnel: [w853] -> w754
            tunnel: [w852] -> w753
            tunnel: [w851] -> w740
            frame #0 {
            }
            frame #1 {
              n249 = call "air pressure setting.vi"() -> ("air pressure indecator"=w852:i32, "deposit speed 2"=w851:dbl)
            }
          }
          n250 = Add(x=w761, y=-2.0) -> (x+y=w772:dbl)
          n251 = call-dynamic "Z Go.vi"("error in (no error)"=w758, "Speed"=5.0, "Position"=w772, "Motion in"=w757) -> ("error out"=w770:errorcluster, "Motion out"=w771:refnum<class "Motion.lvclass">)  [unwired: 6 in]
          n252 = call "Muliti_XY_dispense.vi"("Pressure"=w753, "Path count"=1, "Speed"=w740, "distances"=dbl[][] [[0.0, 194.0], [7.0, 0.0], [0.0, -206.0], [-7.0, 0.0]], "Ultimus V in"=w754, "Motion in"=w771) -> ("Ultimus V out"=w750:refnum<class "Ultimus V2.lvclass">, "Motion out"=w790:refnum<class "Motion.lvclass">)  [unwired: 4 in]
          n253 = flat-sequence {
            tunnel: w750 -> [w846]
            tunnel: [w846] -> w752
            tunnel: w752 -> [w849]
            tunnel: [w849] -> w749
            tunnel: [w848] -> w746
            tunnel: [w847] -> w739
            frame #0 {
            }
            frame #1 {
              n254 = call "air pressure setting.vi"() -> ("air pressure indecator"=w848:i32, "deposit speed 2"=w847:dbl)
            }
          }
          n255 = call-dynamic "wrtCurrent Go.vi"("axis names"=string[] ["X", "Y"], "error in (no error)"=w770, "Speed"=15.0, "distances"=dbl[] [-4.5, -199.0], "Motion in"=w790) -> ("error out"=w765:errorcluster, "Motion out"=w786:refnum<class "Motion.lvclass">)  [unwired: 5 in]
          n256 = call "Muliti_XY_dispense.vi"("Pressure"=w746, "Path count"=4, "Speed"=w739, "distances"=dbl[][] [[0.0, 204.0], [9.0, 0.0], [0.0, -204.0], [-9.0, 0.0]], "Ultimus V in"=w749, "Motion in"=w786) -> ("Ultimus V out"=w748:refnum<class "Ultimus V2.lvclass">, "Motion out"=w780:refnum<class "Motion.lvclass">)  [unwired: 4 in]
          n257 = call-dynamic "wrtCurrent Go.vi"("axis names"=string[] ["X", "Y"], "error in (no error)"=w765, "Speed"=5.0, "distances"=dbl[] [-4.6, -5.0], "Motion in"=w780) -> ("error out"=w764:errorcluster, "Motion out"=w779:refnum<class "Motion.lvclass">)  [unwired: 5 in]
          n258 = flat-sequence {
            tunnel: w748 -> [w842]
            tunnel: [w842] -> w751
            tunnel: w751 -> [w845]
            tunnel: [w845] -> w747
            tunnel: [w844] -> w742
            tunnel: [w843] -> w738
            frame #0 {
            }
            frame #1 {
              n259 = call "air pressure setting.vi"() -> ("air pressure indecator"=w844:i32, "deposit speed 2"=w843:dbl)
            }
          }
          n260 = call "Muliti_XY_dispense.vi"("Pressure"=w742, "Path count"=4, "Speed"=w738, "distances"=dbl[][] [[0.0, 214.0], [18.2, 0.0], [0.0, -214.0], [-18.2, 0.0]], "Ultimus V in"=w747, "Motion in"=w779) -> ("Ultimus V out"=w744:refnum<class "Ultimus V2.lvclass">, "Motion out"=w769:refnum<class "Motion.lvclass">)  [unwired: 4 in]
          n261 = flat-sequence {
            tunnel: w744 -> [w838]
            tunnel: [w838] -> w745
            tunnel: w745 -> [w841]
            tunnel: [w841] -> w743
            tunnel: [w840] -> w741
            tunnel: [w839] -> w737
            frame #0 {
            }
            frame #1 {
              n262 = call "air pressure setting.vi"() -> ("air pressure indecator"=w840:i32, "deposit speed 2"=w839:dbl)
            }
          }
          n263 = call-dynamic "wrtCurrent Go.vi"("axis names"=string[] ["X", "Y"], "error in (no error)"=w764, "Speed"=5.0, "distances"=dbl[] [-4.6, -5.0], "Motion in"=w769) -> ("error out"=w722:errorcluster, "Motion out"=w774:refnum<class "Motion.lvclass">)  [unwired: 5 in]
          n264 = call "Muliti_XY_dispense.vi"("Pressure"=w741, "Path count"=4, "Speed"=w737, "distances"=dbl[][] [[0.0, 224.0], [27.4, 0.0], [0.0, -224.0], [-27.4, 0.0]], "Ultimus V in"=w743, "Motion in"=w774) -> ("Ultimus V out"=w727:refnum<class "Ultimus V2.lvclass">, "Motion out"=w729:refnum<class "Motion.lvclass">)  [unwired: 4 in]
          n265 = flat-sequence {
            tunnel: w729 -> [w803]
            tunnel: [w803] -> w728
            tunnel: w727 -> [w802]
            tunnel: [w802] -> w726
            tunnel: [w801] -> w723
            tunnel: w722 -> [w800]
            tunnel: [w800] -> w721
            tunnel: w728 -> [w810]
            tunnel: w726 -> [w809]
            tunnel: [w808] -> w724
            tunnel: [w807] -> w725
            tunnel: w723 -> [w806]
            tunnel: w721 -> [w805]
            tunnel: [w804] -> w720
            frame #0 {
              n266 = call "redeposit question"() -> ("Do you want to re-depost the chip sides ? 2"=w801:bool)  [unwired: 1 in]
            }
            frame #1 {
              n267 = case shown="True" w806 {
                tunnel: w810 -> [w812 w829]
                tunnel: w809 -> [w813 w832]
                tunnel: [w813 w818] -> w808
                tunnel: [w812 w819] -> w807
                tunnel: w805 -> [w811 w827]
                tunnel: [w811 w821] -> w804
                frame False {
                }
                frame True {
                  n268 = call "Muliti_XY_dispense.vi"("Pressure"=w815, "Path count"=1, "Speed"=w816, "distances"=dbl[][] [[0.0, 224.0], [7.0, 0.0], [0.0, -206.0], [-7.0, 0.0]], "Ultimus V in"=w830, "Motion in"=w829) -> ("Ultimus V out"=w820:refnum<class "Ultimus V2.lvclass">, "Motion out"=w823:refnum<class "Motion.lvclass">)  [unwired: 4 in]
                  n269 = flat-sequence {
                    tunnel: w832 -> [w834]
                    tunnel: [w834] -> w833
                    tunnel: w833 -> [w837]
                    tunnel: [w837] -> w830
                    tunnel: [w836] -> w815
                    tunnel: [w835] -> w816
                    frame #0 {
                    }
                    frame #1 {
                      n270 = call "air pressure setting.vi"() -> ("air pressure indecator"=w836:i32, "deposit speed 2"=w835:dbl)
                    }
                  }
                  n271 = call-dynamic "wrtCurrent Go.vi"("axis names"=string[] ["X", "Y"], "error in (no error)"=w827, "Speed"=15.0, "distances"=dbl[] [27.4, 0.0], "Motion in"=w823) -> ("error out"=w821:errorcluster, "Motion out"=w822:refnum<class "Motion.lvclass">)  [unwired: 5 in]
                  n272 = call "Muliti_XY_dispense.vi"("Pressure"=w815, "Path count"=1, "Speed"=w816, "distances"=dbl[][] [[0.0, -224.0], [7.0, 0.0], [0.0, -206.0], [-7.0, 0.0]], "Ultimus V in"=w820, "Motion in"=w822) -> ("Ultimus V out"=w818:refnum<class "Ultimus V2.lvclass">, "Motion out"=w819:refnum<class "Motion.lvclass">)  [unwired: 4 in]
                }
              }
            }
          }
        }
        n273 = call "XYZTheta Go.vi"("error in (no error)"=w648, "XYZTheta In"=dbl[] [500.0, 1000.0, 0.0, 0.1], "Motion in"=w669) -> ("error out"=w679:errorcluster, "Motion out"=w677:refnum<class "Motion.lvclass">)  [unwired: 6 in, 1 out]
        n274 = call "Display Message to User3"("error in (no error)"=w679) -> ()  [unwired: 9 in, 2 out]
        n275 = call-dynamic "Disconnect.vi"("Ultimus V in"=w668) -> ()  [unwired: 9 in, 1 out]
      }
      event "Needle Alignment": Value Change {
        (unwired) "Needle Alignment in progress ...." ("String")
        # "CF height"
        # "surface z offset"
        # "first needle park position\nneedle gap on Z value : 0.5 mm"
        # "Syringe-camera offset"
        n276 = event-data() -> ()  [unwired: 1 in, 6 out]
        n277 = Array Subset(array=w866, index (row)=0, length (row)=1 ("length")) -> (w869:dbl[][])  [unwired: 2 in]
        n278 = Reshape Array(w869, 4 ("dimension size")) -> (w868:dbl[])
        n279 = Index Array(array=w868, index=2) -> (element=w865:dbl)
        n280 = call-poly <vilib>:"Read Delimited Spreadsheet.vi"("file path (dialog if empty)"=path "D:/INTT/V1/Assembly Data/Tool Offsets/Dispense Tip Offset.txt", "number of rows (all:-1)"=-1) -> ("first row"=w916:dbl[])  [unwired: 8 in, 5 out]
        n281 = Index Array(array=w916, index #1=0 ("index"), index #2=1 ("index")) -> (element #1=w911:dbl, element #2=w910:dbl)
        n282 = Add(x=14.2 ("element"), y=w874) -> (x+y=w876:dbl)
        n283 = Add(x=w865, y=w876) -> (x+y=w875:dbl)
        n284 = Build Array(424.448, 1040.76, w875, 0.0 ("element")) -> (w873:dbl[])
        n285 = Build Array(w911, w910, 0.0 ("element"), 0.0 ("element")) -> (w885:dbl[])
        n286 = call "XYZTheta Go.vi"("XYZTheta In"=w873, "Motion in"=w900) -> ("error out"=w909:errorcluster, "XYZTheta Out"=w890:dbl[], "Motion out"=w899:refnum<class "Motion.lvclass">)  [unwired: 7 in]
        n287 = call "Display Message to User10"("error in (no error)"=w909) -> ("error out"=w906:errorcluster)  [unwired: 9 in, 1 out]
        n288 = call-dynamic "Z Go.vi"("error in (no error)"=w906, "Speed"=20.0, "Position"=0.0, "Motion in"=w899) -> ("Motion out"=w898:refnum<class "Motion.lvclass">)  [unwired: 6 in, 1 out]
        n289 = Replace Array Subset(array=w890, new element=0.0 ("new element/subarray"), index=2) -> (w887:dbl[])
        n290 = call "Joystick and Camera SHIH VPC- external Connection.vi"("Motion in"=w898, "XYZTheta"=w887, "Measurement Point"="Touch Needle on a surface") -> ("Motion out"=w896:refnum<class "Motion.lvclass">, "Gantry"=w886:dbl[])  [unwired: 4 in, 2 out]
        n291 = Subtract(x=w886, y=w885) -> (x-y=w884:dbl[])
        n292 = call "Joystick and Camera SHIH VPC- external Connection.vi"("Motion in"=w896, "XYZTheta"=w884, "Measurement Point"="Measure the touch spot with camera") -> ("Motion out"=w892:refnum<class "Motion.lvclass">, "Gantry"=w895:dbl[])  [unwired: 4 in, 2 out]
        n293 = Subtract(x=w886, y=w895) -> (x-y=w894:dbl[])
        n294 = call-poly <vilib>:"Write Delimited Spreadsheet.vi"("file path (dialog if empty)"=path "D:/INTT/V1/Assembly Data/Tool Offsets/Dispense Tip Offset.txt", "1D data"=w894, "append to file? (new file:F)"=FALSE) -> ()  [unwired: 11 in, 2 out]
      }
      event "Pick and place": Value Change {
        (unwired) "PICK and PLACE samples ..." ("String")
        n295 = event-data() -> ()  [unwired: 1 in, 6 out]
        n296 = Build Array(0.0 ("element"), 0.0 ("element"), 0.0 ("element"), 0.0 ("element")) -> (w934:dbl[])
        n297 = Build Array(0.0 ("element"), 0.0 ("element"), 0.0 ("element"), 0.0 ("element")) -> (w933:dbl[])
        n298 = case shown="False" w928 {
          tunnel: w953 -> [w1119 w1141]
          tunnel: [w1118 w1140] -> _
          frame False {
            n299 = Array Subset(array=w1119, index (row)=0 ("index"), length (row)=1 ("length")) -> (w1121:dbl[][])  [unwired: 2 in]
            n300 = Build Array(11.75 ("element"), 173.55 ("element"), 0.0 ("element"), 0.0 ("element")) -> (w1125:dbl[])
            n301 = Reshape Array(w1121, 4 ("dimension size")) -> (w1120:dbl[])
            n302 = Add(x=w1125, y=w1120) -> (x+y=w1118:dbl[])
          }
          frame True {
            n303 = Array Subset(array=w1141, index (row)=0 ("index"), length (row)=1 ("length")) -> (w1131:dbl[][])  [unwired: 2 in]
            n304 = Build Array(11.75 ("element"), 56.85 ("element"), 0.0 ("element"), 0.0 ("element")) -> (w1135:dbl[])
            n305 = Reshape Array(w1131, 4 ("dimension size")) -> (w1130:dbl[])
            n306 = Add(x=w1135, y=w1130) -> (x+y=w1140:dbl[])
          }
        }
        n307 = Not(x=w928) -> (.not. x?=w927:bool)
        n308 = case shown="True" w927 {
          tunnel: w934 -> [w1112 w1115]
          tunnel: w933 -> [w1113 w1116]
          tunnel: [w1114 w1117] -> w932
          frame False {
            n309 = Build Array(w1113, w1112) -> (w1114:dbl[][])
          }
          frame True {
            n310 = Build Array(w1115, w1116) -> (w1117:dbl[][])
          }
        }
        n311 = Add(x=1.0, y=w924) -> (x+y=w920:dbl)
        n312 = Quotient & Remainder(x=w920, y=2.0) -> (x-y*floor(x/y)=w922:dbl)  [unwired: 1 out]
        n313 = Equal To 0?(x=w922) -> (x = 0?=w921:bool)
        n314 = for {
          tunnel: [w977] -> w926
          tunnel: w932 -> [w976] mode=indexing
          tunnel: w929 -> [w973] mode=indexing
          n315 = Index Array(array=w973, index=3) -> (element=w974:dbl)
          n316 = Multiply(x=w974, y=-1.0) -> (x*y=w972:dbl)
          n317 = Index Array(array=w976, index=0) -> (element=w983:dbl)
          n318 = Index Array(array=w976, index=1) -> (element=w982:dbl)
          n319 = call-poly <vilib>:"2D Cartesian Coordinate Rotation.vi"("theta"=w972, "y"=w982, "x"=w983) -> ("y out"=w985:dbl, "x out"=w984:dbl)  [unwired: 6 in, 1 out]
          n320 = Build Array(w984, w985, 0.0 ("element"), 0.0 ("element")) -> (w977:dbl[])
        }
        "?" <- w926
        n321 = Array Subset(array=w929, index (row)=0 ("index"), length (row)=1 ("length")) -> (w940:dbl[][])  [unwired: 2 in]
        n322 = Reshape Array(w940, 4 ("dimension size")) -> (w931:dbl[])
        n323 = Add(x=w926, y=w931) -> (x+y=w930:dbl[])
        "CT sum up" <- w930
        n324 = call-poly <vilib>:"Read Delimited Spreadsheet.vi"("file path (dialog if empty)"=path "D:/INTT/V1/Assembly Data/Tool Offsets/Bellows Tool Offset.txt", "number of rows (all:-1)"=-1) -> ("first row"=w968:dbl[])  [unwired: 8 in, 5 out]
        n325 = Index Array(array=w968, index #1=0 ("index"), index #2=1 ("index"), index #3=2 ("index")) -> (element #1=w964:dbl, element #2=w963:dbl, element #3=w962:dbl)
        n326 = for {
          N: 1 -> [_]
          tunnel: w971 -> [w1001]
          tunnel: [w1021] -> w961
          tunnel: w960 -> [w995] mode=indexing
          tunnel: [w1009] -> w956
          tunnel: w957 -> [w1000]
          tunnel: w964 -> [w1023]
          tunnel: w963 -> [w1022]
          tunnel: w962 -> [w1020]
          tunnel: w949 -> [w1015]
          tunnel: w955 -> [w1003]
          tunnel: w930 -> [w1002]
          tunnel: w951 -> [w998]
          tunnel: w929 -> [w994]
          tunnel: w926 -> [w993]
          tunnel: w921 -> [w992]
          w1011 = 0 ("Write")
          w1014 = TRUE ("Write Value")
          # "putback pickup tool"
          # "pickup tool"
          # "pickup tool height offset"
          # "Pick up PICKUP TOOL"
          # "Pick up CHIPs/Sensor and place on HDI"
          n327 = Build Array(w1023, w1022, w1020, 0.0 ("element")) -> (w996:dbl[])
          n328 = Add(x=w995, y=w996) -> (x+y=w990:dbl[])
          n329 = call "XYZTheta-2Zspeed Go.vi"("XYZTheta In"=w990, "Motion in"=w1001) -> ("error out"=w999:errorcluster, "Motion out"=w997:refnum<class "Motion.lvclass">)  [unwired: 7 in, 1 out]
          n330 = call "WriteReadWait.vi"("Read Value"=w1014, "Write Value"=w1014, "error in (no error)"=w999, "Read"=w1011, "Write"=w1011, "I-O in"=w1000) -> ("error out"=w1013:errorcluster, "I-O out"=w1012:refnum<class "NI-DAQ.lvclass">)  [unwired: 4 in]
          n331 = Replace Array Subset(array=w996, new element=-16.0 ("t"), index=2) -> (w1018:dbl[])
          n332 = for {
            N: w1015 -> [_]
            tunnel: w997 -> [w1053]
            tunnel: w1018 -> [w1052]
            tunnel: w1013 -> [w1051]
            tunnel: [w1050] -> w1024
            tunnel: w1012 -> [w1049]
            tunnel: [w1048] -> w1010
            tunnel: [w1047] -> w1017
            tunnel: w1003 -> [w1044]
            tunnel: w1002 -> [w1041]
            tunnel: w998 -> [w1043] mode=indexing
            tunnel: w994 -> [w1042] mode=indexing
            tunnel: w993 -> [w1040]
            tunnel: [w1038] -> w989 mode=concatenating
            n333 = flat-sequence {
              tunnel: [w1076] -> w1054
              tunnel: w1053 -> [w1075]
              tunnel: w1052 -> [w1074]
              tunnel: w1051 -> [w1072]
              tunnel: w1049 -> [w1066]
              tunnel: [w1071] -> w1046
              tunnel: [w1059] -> w1045
              tunnel: w1044 -> [w1058]
              tunnel: w1041 -> [w1069]
              tunnel: [w1060] -> _
              tunnel: w1040 -> [w1060]
              tunnel: [w1060] -> w1039
              tunnel: w1054 -> [w1102]
              tunnel: [w1111] -> w1050
              tunnel: [w1110] -> _
              tunnel: [w1106] -> w1048
              tunnel: [w1083] -> w1047
              tunnel: w1046 -> [w1108]
              tunnel: w1045 -> [w1104]
              tunnel: w1043 -> [w1105]
              tunnel: w1042 -> [_]
              tunnel: w1041 -> [w1084]
              tunnel: w1039 -> [_]
              tunnel: [w1077] -> w1038
              frame #0 {
                w1064 = FALSE ("Write Value")
                w1070 = TRUE ("Write Value")
                w1057 = 1 ("Write")
                # "pickup module"
                # "release module"
                # "pickup sample from tray"
                n334 = Add(x=w1069, y=w1074) -> (x+y=w1073:dbl[])
                n335 = call "XYZTheta-2Zspeed Go.vi"("error in (no error)"=w1072, "XYZTheta In"=w1073, "Motion in"=w1075) -> ("error out"=w1067:errorcluster, "Motion out"=w1076:refnum<class "Motion.lvclass">)  [unwired: 6 in, 1 out]
                n336 = call "Time Delay"("error in (no error)"=w1067) -> ("error out"=w1061:errorcluster)  [unwired: 10 in]
                n337 = call "0"("error in (no error)"=w1061) -> ("error out"=w1062:errorcluster)  [unwired: 9 in, 1 out]
                n338 = call "WriteReadWait.vi"("Read Value"=w1064, "Write Value"=w1064, "error in (no error)"=w1062, "Read"=w1058, "Write"=w1058, "I-O in"=w1066) -> ("error out"=w1063:errorcluster, "I-O out"=w1065:refnum<class "NI-DAQ.lvclass">)  [unwired: 4 in]
                n339 = call "Time Delay3"("error in (no error)"=w1063) -> ("error out"=w1068:errorcluster)  [unwired: 10 in]
                n340 = call "WriteReadWait.vi"("Read Value"=w1070, "Write Value"=w1070, "error in (no error)"=w1068, "Read"=w1057, "Write"=w1057, "I-O in"=w1065) -> ("error out"=w1056:errorcluster, "I-O out"=w1071:refnum<class "NI-DAQ.lvclass">)  [unwired: 4 in]
                n341 = call "release"("error in (no error)"=w1056) -> ("error out"=w1055:errorcluster)  [unwired: 9 in, 1 out]
                n342 = call "Delay5"("error in (no error)"=w1055) -> ("error out"=w1059:errorcluster)  [unwired: 10 in]
              }
              frame #1 {
                w1107 = 1 ("Write")
                w1109 = FALSE ("Write Value")
                # "7mins"
                # "lift for chip/sensor thickness"
                # "place sample on HDI"
                n343 = Add(x=w1105, y=dbl[] [0.0, 0.0, -16.0, 0.0]) -> (x+y=w1100:dbl[])
                n344 = call-dynamic "Get Current Position.vi"("Motion in"=w1102) -> ("XYZTheta Out"=w1098:dbl[], "Motion out"=w1101:refnum<class "Motion.lvclass">)  [unwired: 8 in, 1 out]
                "gantry position test" <- w1098
                n345 = Array Subset(array=w1084, index=0, length=2) -> (w1087:dbl[])
                n346 = Build Array (concatenate)(w1087, 0.0 ("element"), 0.0 ("element")) -> (w1086:dbl[])
                n347 = Subtract(x=w1100, y=w1086) -> (x-y=w1099:dbl[])
                "displacement" <- w1099
                n348 = Array Subset(array=w1098, index=0, length=2) -> (w1093:dbl[])
                n349 = Build Array (concatenate)(w1093, 0.0 ("element"), 0.0 ("element")) -> (w1092:dbl[])
                n350 = Add(x=w1092, y=w1099) -> (x+y=w1081:dbl[])
                n351 = Add(x="offset", y=w1081) -> (x+y=w1077:dbl[])
                "gantry target position" <- w1077
                n352 = call "XYZTheta-2Zspeed Go.vi"("error in (no error)"=w1104, "XYZTheta In"=w1077, "Motion in"=w1101) -> ("error out"=w1103:errorcluster, "XYZTheta Out"=w1110:dbl[], "Motion out"=w1111:refnum<class "Motion.lvclass">)  [unwired: 6 in]
                n353 = call "1"("error in (no error)"=w1103) -> ("error out"=w1080:errorcluster)  [unwired: 9 in, 1 out]
                n354 = call "WriteReadWait.vi"("Read Value"=w1109, "Write Value"=w1109, "error in (no error)"=w1080, "Read"=w1107, "Write"=w1107, "I-O in"=w1108) -> ("error out"=w1079:errorcluster, "I-O out"=w1106:refnum<class "NI-DAQ.lvclass">)  [unwired: 4 in]
                n355 = call "Time Delay6"("error in (no error)"=w1079) -> ("error out"=w1078:errorcluster)  [unwired: 10 in]
                n356 = call "Time Delay4"("error in (no error)"=w1078) -> ("error out"=w1083:errorcluster)  [unwired: 10 in]
              }
            }
          }
          n357 = case shown="True" w992 {
            tunnel: [dbl[] [346.77, 628.513, 53.0078, 0.0] w1037] -> w991
            tunnel: w990 -> [_ w1037]
            tunnel: w989 -> [w1031 w1035]
            frame False {
              # "north side"
              n358 = call-poly <vilib>:"Write Delimited Spreadsheet.vi"("file path (dialog if empty)"=path "D:/INTT/V1/Assembly Data/ladder assembly/northtool.txt" ("file path (dialog if empty) 4"), "format (%.3f)"="%.10f", "1D data"=w1031) -> ()  [unwired: 11 in, 2 out]
            }
            frame True {
              # "south side"
              n359 = call-poly <vilib>:"Write Delimited Spreadsheet.vi"("file path (dialog if empty)"=path "D:/INTT/V1/Assembly Data/ladder assembly/southtool.txt" ("file path (dialog if empty) 4"), "format (%.3f)"="%.10f", "1D data"=w1035) -> ()  [unwired: 11 in, 2 out]
            }
          }
          n360 = call "XYZTheta-2Zspeed Go.vi"("error in (no error)"=w1017, "XYZTheta In"=w991, "Motion in"=w1024) -> ("error out"=w1006:errorcluster, "Motion out"=w1028:refnum<class "Motion.lvclass">)  [unwired: 6 in, 1 out]
          n361 = call "Time Delay9"("error in (no error)"=w1006) -> ("error out"=w988:errorcluster)  [unwired: 10 in]
          n362 = call "?"("error in (no error)"=w988) -> ("error out"=w987:errorcluster)  [unwired: 9 in, 1 out]
          n363 = call-dynamic "Digital Write 1 Channel.vi"("DAQ Module"=0, "error constant"=w987, "Value"=FALSE, "Channel"=0, "NI-DAQ.lvclass"=w1010) -> ("error IO"=w1007:errorcluster, "NI-DAQ.lvclass 2"=w1009:refnum<class "NI-DAQ.lvclass">)  [unwired: 5 in]
          n364 = call "Time Delay10"("error in (no error)"=w1007) -> ("error out"=w1025:errorcluster)  [unwired: 10 in]
          n365 = call-dynamic "Z Go.vi"("error in (no error)"=w1025, "Speed"=10.0, "Position"=0.0 ("new element/subarray"), "Motion in"=w1028) -> ("Motion out"=w1021:refnum<class "Motion.lvclass">)  [unwired: 6 in, 1 out]
        }
      }
      event "GOTO": Value Change {
        (unwired) "GOING to a position" ("String")
        n366 = event-data() -> ()  [unwired: 1 in, 6 out]
        n367 = call "XYZTheta Go.vi"("XYZTheta In"="Parking position", "Motion in"=w1149) -> ("Motion out"=w1147:refnum<class "Motion.lvclass">)  [unwired: 7 in, 2 out]
      }
      event "READ Position": Value Change {
        n368 = event-data() -> ()  [unwired: 1 in, 6 out]
        n369 = call-dynamic "Get Current Position.vi"("Motion in"=w1169) -> ("XYZTheta Out"=→"Gantry current position":dbl[], "Motion out"=w1168:refnum<class "Motion.lvclass">)  [unwired: 8 in, 1 out]
      }
      event "HDI vacuum": Value Change {
        n370 = event-data() -> ()  [unwired: 1 in, 6 out]
        n371 = call "WriteReadWait.vi"("Read Value"="vacuum", "Write Value"="vacuum", "Read"=w1182, "Write"=w1182, "I-O in"=w1185) -> ("error out"=w1183:errorcluster, "I-O out"=w1172:refnum<class "NI-DAQ.lvclass">)  [unwired: 5 in]
        n372 = call "Time Delay2"("error in (no error)"=w1183) -> ()  [unwired: 10 in, 1 out]
      }
      event Timeout {
        n373 = event-data() -> ()  [unwired: 1 in, 3 out]
        n374 = call-dynamic "Digital Read 1 Channel.vi"("Read"=w1198, "NI-DAQ in"=w1199) -> ("Value"=→"Status":bool, "NI-DAQ out"=w1197:refnum<class "NI-DAQ.lvclass">)  [unwired: 7 in, 1 out]
      }
    }
    "Measured HDI size" <- w28
    "MPT positions on stave" <- w29
    "Stave mark" <- w27
    "measured HDI top-left position" <- w24
    n375 = feedback-in #1(w28) -> ()
    n376 = feedback-in #2(w27) -> ()
    n377 = feedback-in #3(w24) -> ()
    n378 = feedback-in #4(w13) -> ()
    n379 = feedback-in #5(w39) -> ()
    n380 = feedback-in #6(w36) -> ()
    n381 = feedback-in #7(w44) -> ()
    n382 = feedback-in #8(w29) -> ()
    n383 = feedback-in #9(w45) -> ()
    "# of tasks excuted" <- w41
  }
  n384 = call-dynamic "Disconnect.vi"("Controller in"=w5) -> ()  [unwired: 9 in, 1 out]
  n385 = call-dynamic "Disconnect.vi"("I-O in"=w2) -> ()  [unwired: 9 in, 1 out]
